vi "SpectrometerSpinCoater_v01.vi"() -> ()   [LabVIEW 2018]
uses:
  <instrlib>/Classes/CCD/Abstract_CCD/Abstract_CCD.lvclass
  TypDef/DeviceQueue_TypeDef.ctl
  TypDef/DeviceQueue_Action.ctl
  TypDef/DataQueue_TypeDef.ctl
  TypDef/DataQueue_Action.ctl
  <vilib>/Utility/error.llb/DialogType.ctl
  <instrlib>/Classes/CCD/Avantes/Avantes.lvclass
  C:/Program Files/National Instruments/LabVIEW 2018/instr.lib/Classes/CCD/Abstract_CCD/Abstract_CCD.lvclass
  <vilib>/Instr/_visa.llb/VISA Configure Serial Port (Instr).vi
panel:
  out "Arduino":bool
  out "NKT":bool
  out "Spectromter":bool
  in  "Abort Button":bool
  in  "Stop Button":bool
  in  "Tab Control":enum32{"Measure", "Settings"}(tab)
  out "Action":string
  in  "Preview":bool
  out "XY Graph":T1(graph)
  in  "Frames for Dark/Ref":dbl=1.0
  in  "StartSpin_Button":bool
  out "Overall Time":dbl
  in  "Seconds after Spin Stop":dbl[unit]=0.5
  in  "Program Spin Coater\nSpeed (rpm)          Time (s)":dbl[][](array[numeric])
  in  "Record RefSpec":bool
  in  "Record_Darkspec":bool
  in  "Comments":string="Just for testing"
  in  "File Name":string="Temp"
  in  "Save Path":path=path "C:/Users/Timo/Desktop/SpinCoater/Measurement"
  in  "Seconds to Spin Start":dbl[unit]=1.0
  in  "Calculate Frames":bool=TRUE
  in  "Frames":i32
  out "Frame Rate":dbl[unit]
  in  "Integration Time":dbl[unit]=3e-05
  in  "StartMeasurement_Button":bool
  in  "Speed":dbl
  in  "Milliseconds":dbl
  in  "Debug":bool
  in  "Port Arduino":refnum<visa-resource-name>="COM3"
  out "Error Arduino":bool caption="Error"
  in  "Init_Arduino":bool=TRUE caption="Init"
  out "Caption_Settings_Arduino":string="Arduino"
  out "Caption_Settings_NKT":string="NKT Laser"
  out "Error_Spectromter":bool caption="Error"
  in  "Init_Spectrometer":bool=TRUE caption="Init"
  out "Caption_Settings_Spectrometer":string="Spectromter"
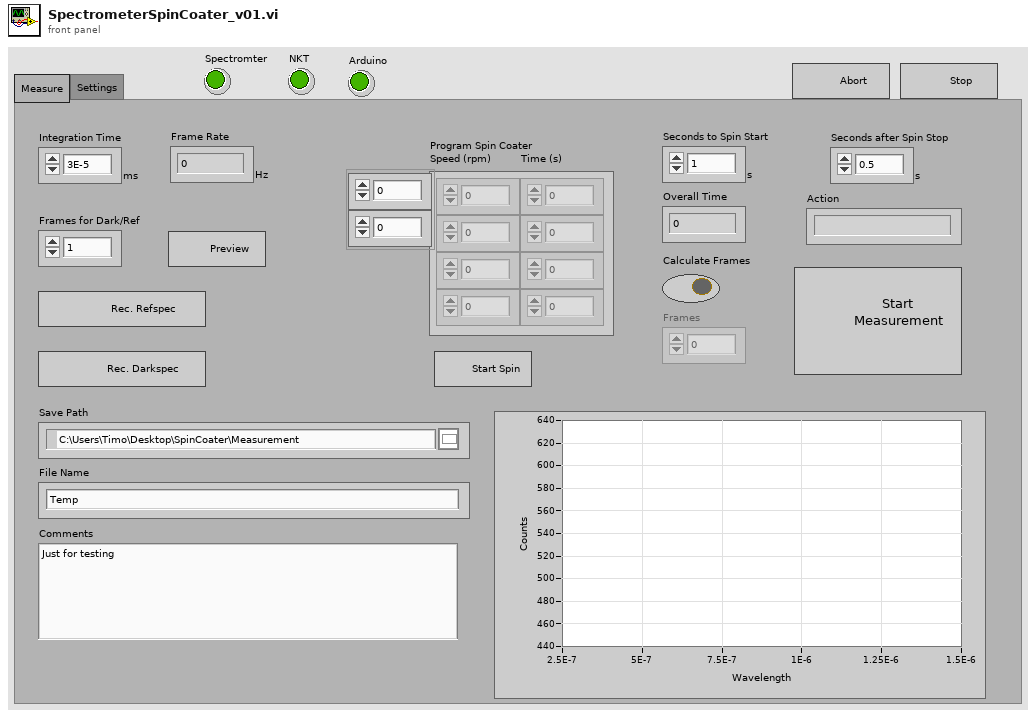
[diagram p1: front panel]
types:
  T1 = cluster{"Wavlength":dbl[unit][], "Image":dbl[]}[]
  T2 = cluster{"Dark":cluster{"Image":dbl[][][], "Frame Size":cluster{"F":i32, "Y":i32, "X":i32}}[], "Ref":cluster{"Image":dbl[][][], "Frame Size":cluster{"F":i32, "Y":i32, "X":i32}}[], "Wavlength":dbl[unit][], "spec":dbl[][]}
  T3 = cluster{"Port Arduino":refnum<visa-resource-name>, "Abstract_CCD.lvclass":refnum<class "Abstract_CCD.lvclass">}
  T4 = typedef "DataQueue_TypeDef.ctl" = cluster{"QueueAction":T5, "Data":cluster{"Image":dbl[][][], "Frame Size":cluster{"F":i32, "Y":i32, "X":i32}}[], "Data_Raw":cluster{"Image":dbl[][][], "Frame Size":cluster{"F":i32, "Y":i32, "X":i32}}[], "Data_Dark":cluster{"Image":dbl[][][], "Frame Size":cluster{"F":i32, "Y":i32, "X":i32}}[], "Data_Ref":cluster{"Image":dbl[][][], "Frame Size":cluster{"F":i32, "Y":i32, "X":i32}}[], "Device Information":string[], "Numeric Control":dbl, "Boolean":bool, "Wavelength":dbl[unit][], "Time":dbl[], "Time Stamp":timestamp}
  T5 = typedef "DataQueue_Action.ctl" = enum16{"TimeOut", "Close_Program", "Measure_InSituSpinCoating", "Save_Data", "Set_Ref", "Set_Dark", "Set_Wavelength", "Spectrometer_Measure"}
  T6 = typedef "DeviceQueue_TypeDef.ctl" = cluster{"QueueAction":T7, "Numeric 1":dbl, "Numeric 2":dbl, "Boolean 1":bool, "Boolean 2":bool, "Spin Program":dbl[][]}
  T7 = typedef "DeviceQueue_Action.ctl" = enum16{"TimeOut", "Close_Program", "Abort", "Spectrometer_Init", "Spectrometer_Close", "Spectrometer_Measure", "Spectrometer_Preview", "Spectrometer_Abort", "Spectrometer_SetIntegrationTime", "Spectrometer_SetFrames", "Spectrometer_SetDarkspec", "Spectrometer_SetReference", "Laser_Init", "Laser_Close", "Arduino_Init", "Arduino_Close", "Arduino_LoadProgram", "Arduino_StartProgram", "Arduino_SetSpeed", "Arduino_SetMillis", "Arduino_StopSpin", "Measure_InSitu"}
  T8 = cluster{"Image":dbl[][][], "Frame Size":cluster{"F":i32, "Y":i32, "X":i32}}[]
  T9 = cluster{"Image":dbl[][][], "Frame Size":cluster{"F":i32, "Y":i32, "X":i32}}
  T10 = cluster{u32, u32, u32, "spec":dbl[][], "Image":dbl[], "Image":dbl[], dbl[], "Time":dbl[], "Numeric Control":dbl}
  T11 = typedef "DialogType.ctl" = u16
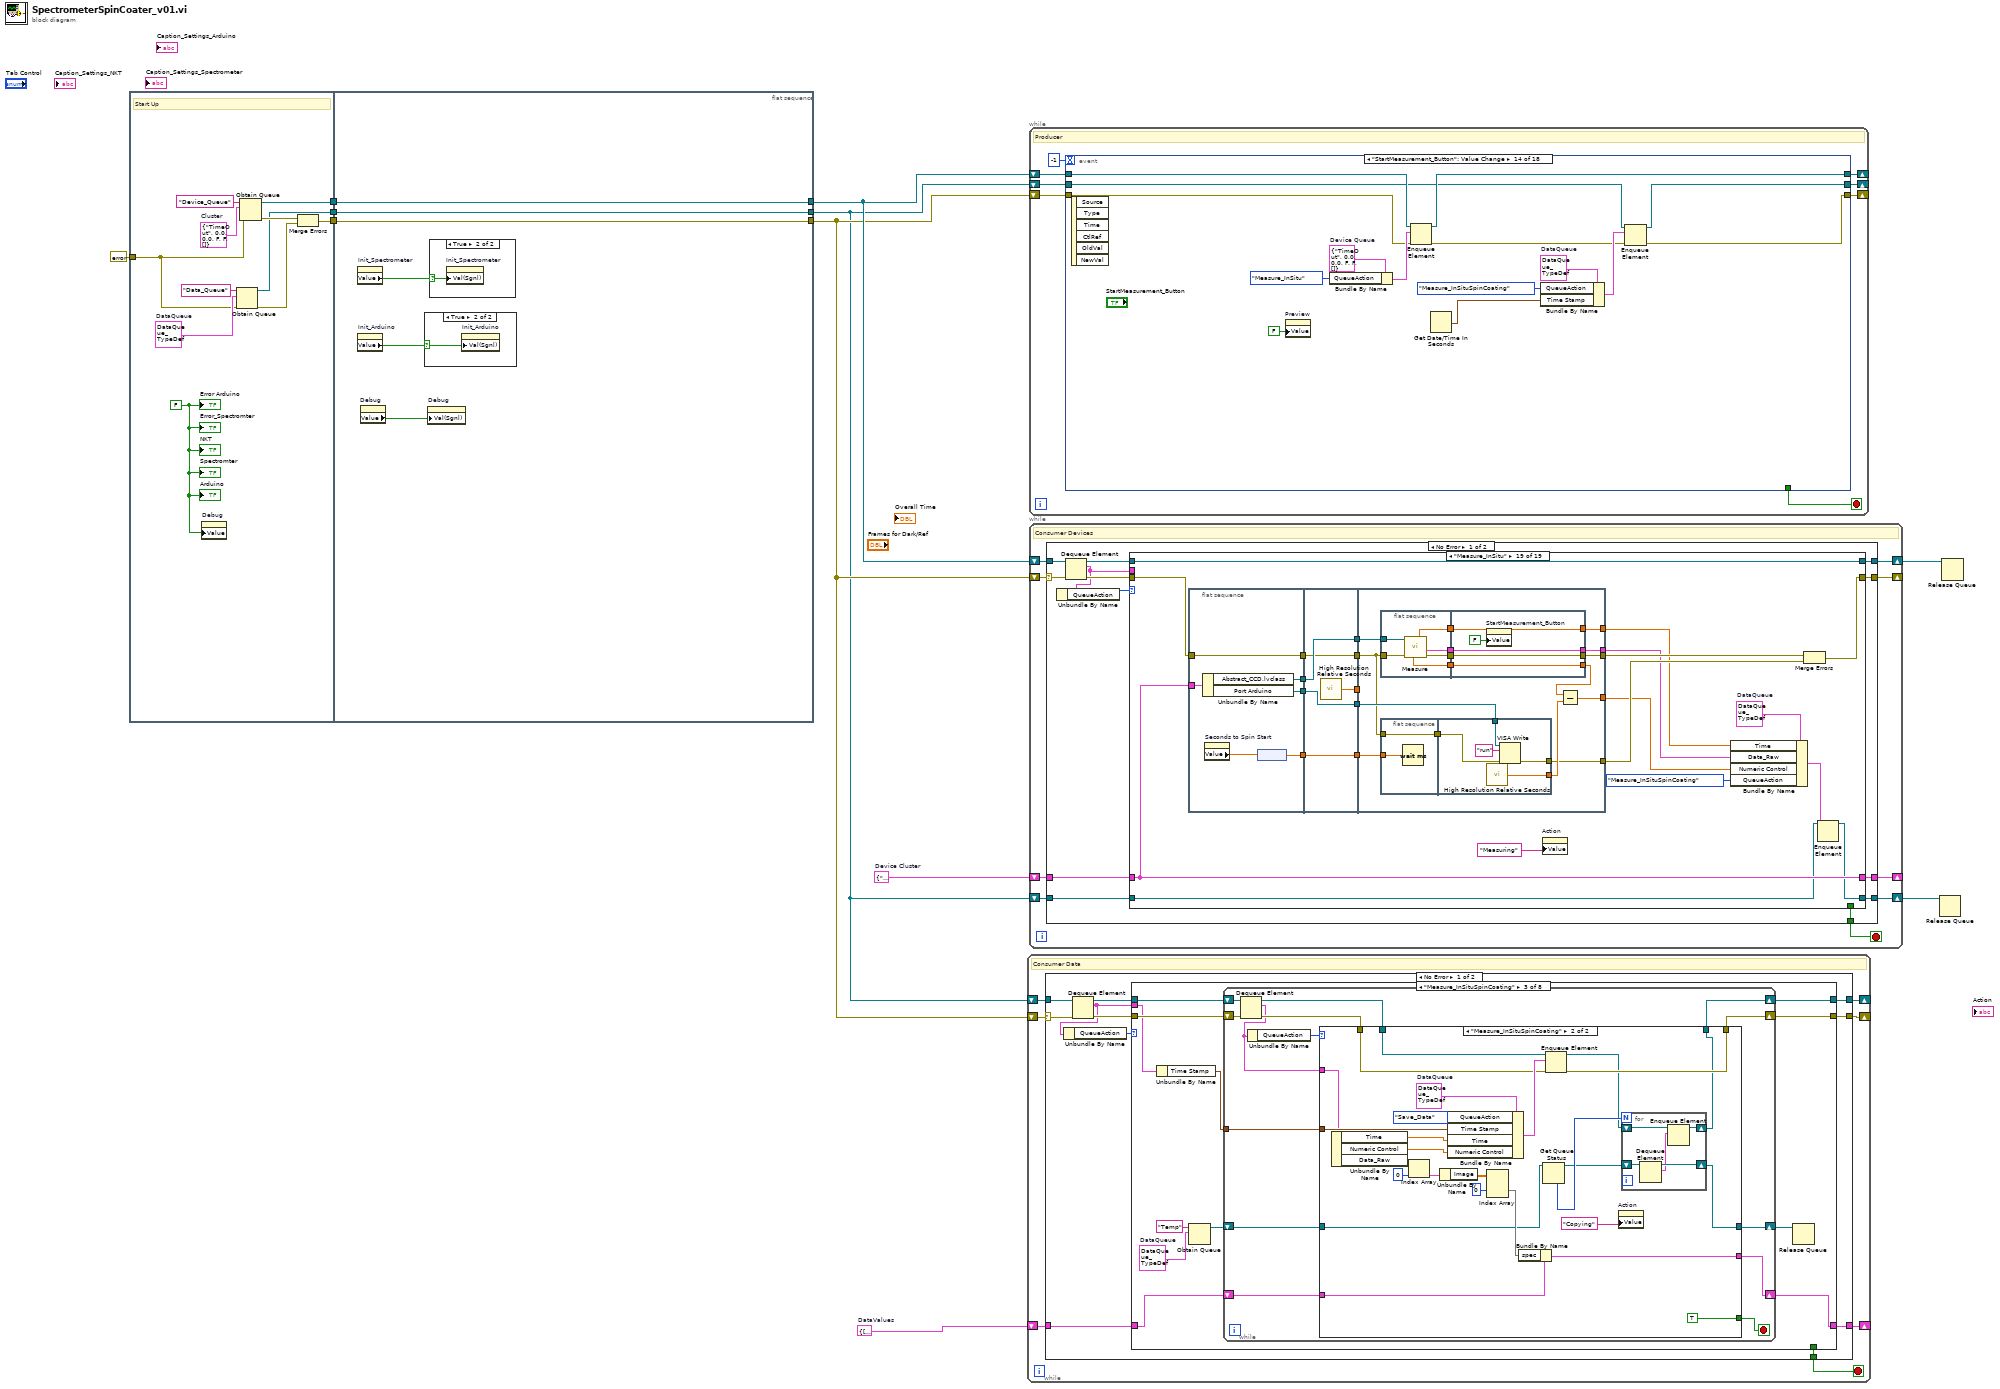
[diagram p0: block diagram]
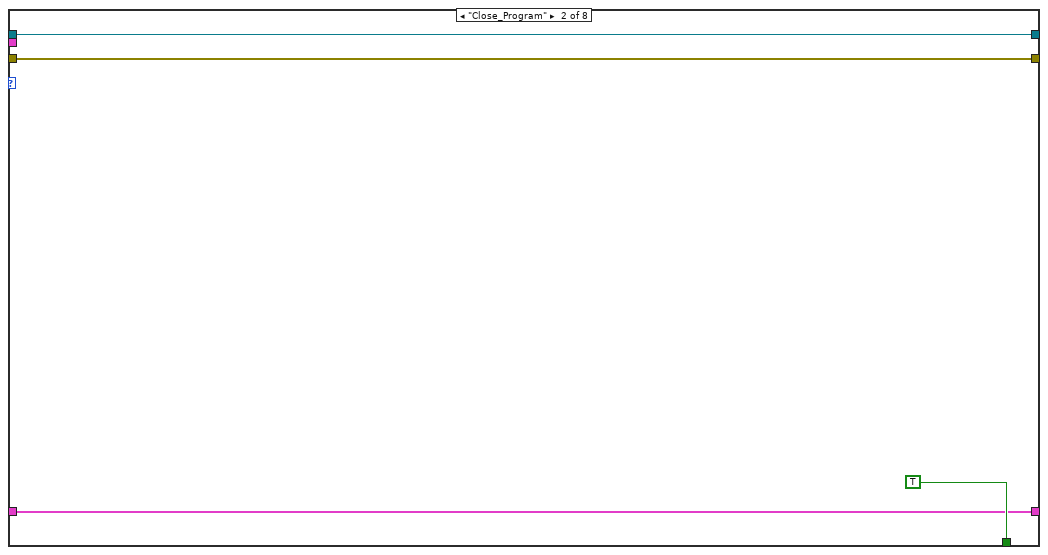
[diagram p5: hidden frame]
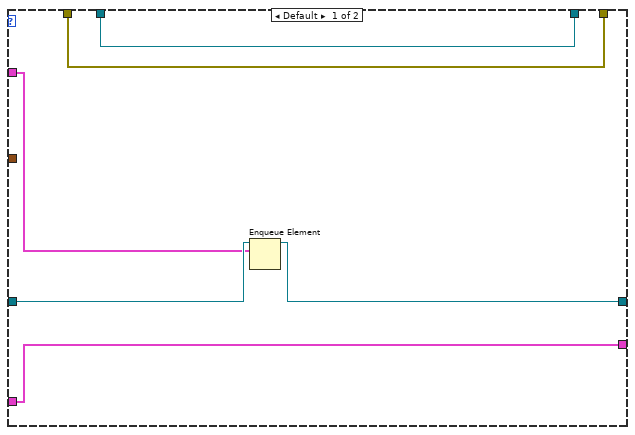
[diagram p6: hidden frame]
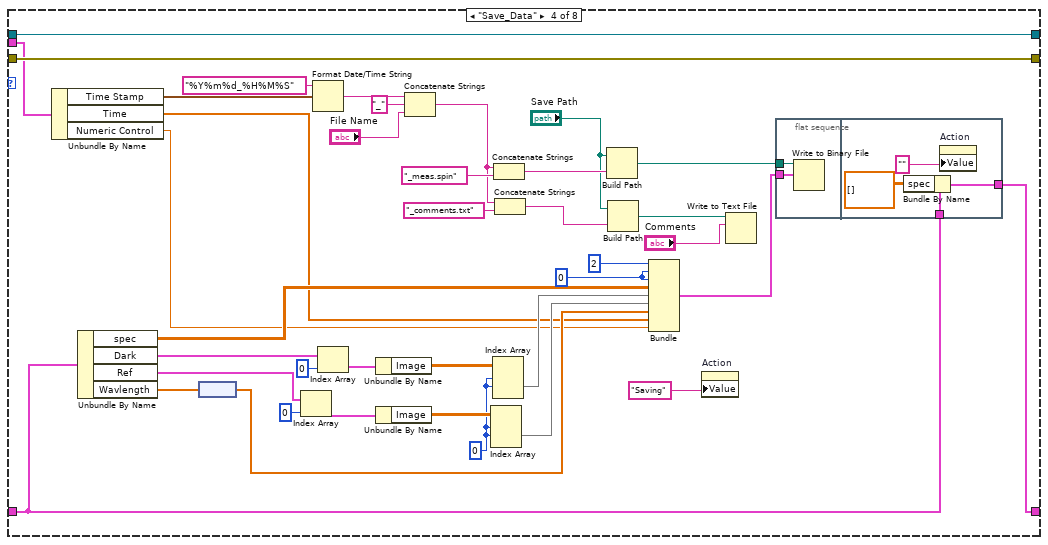
[diagram p7: hidden frame]
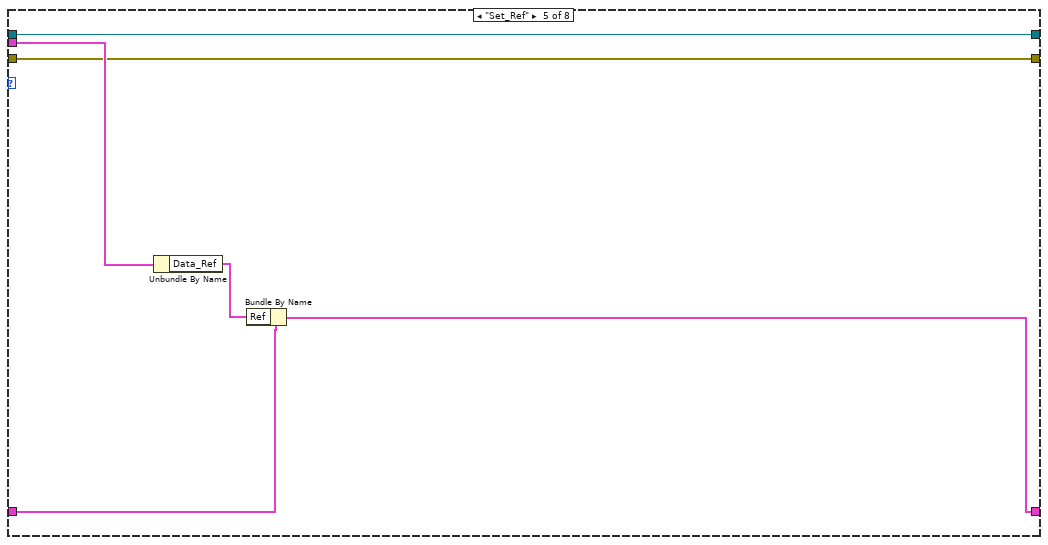
[diagram p8: hidden frame]
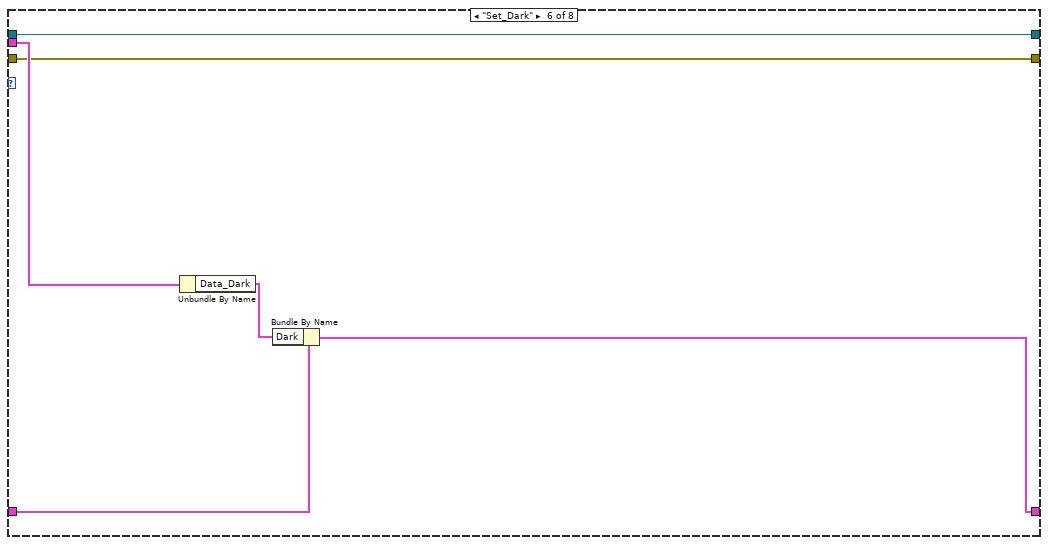
[diagram p9: hidden frame]
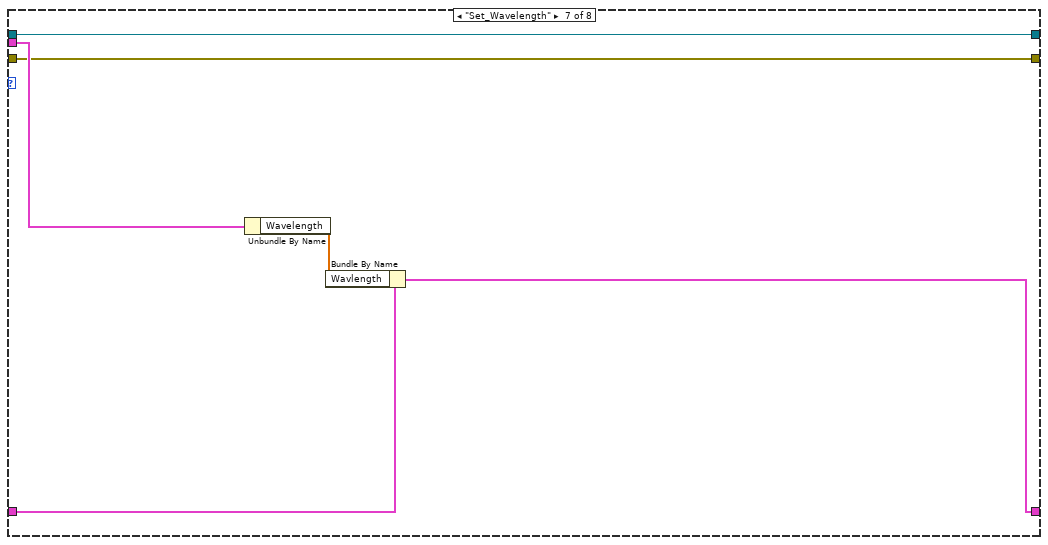
[diagram p10: hidden frame]
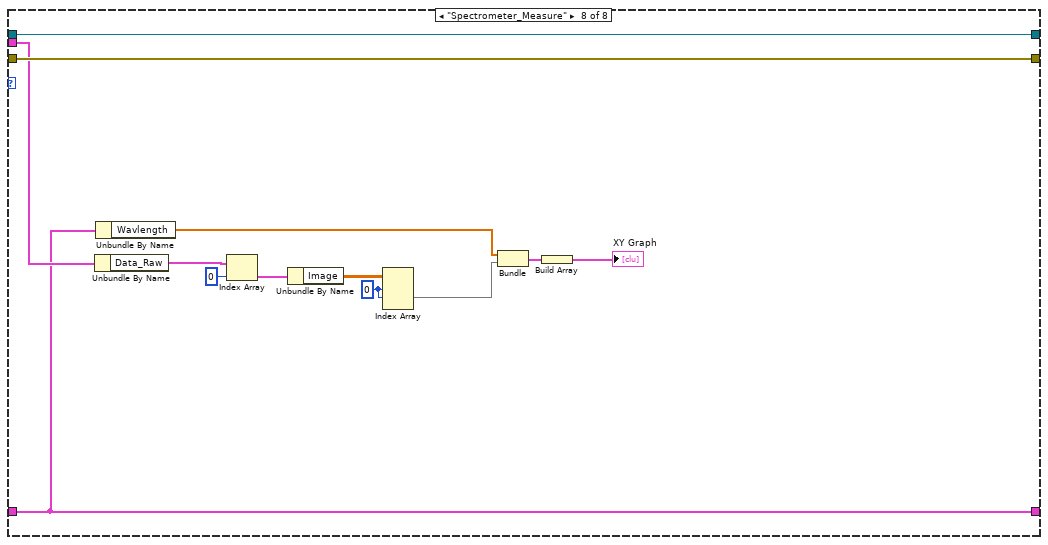
[diagram p11: hidden frame]
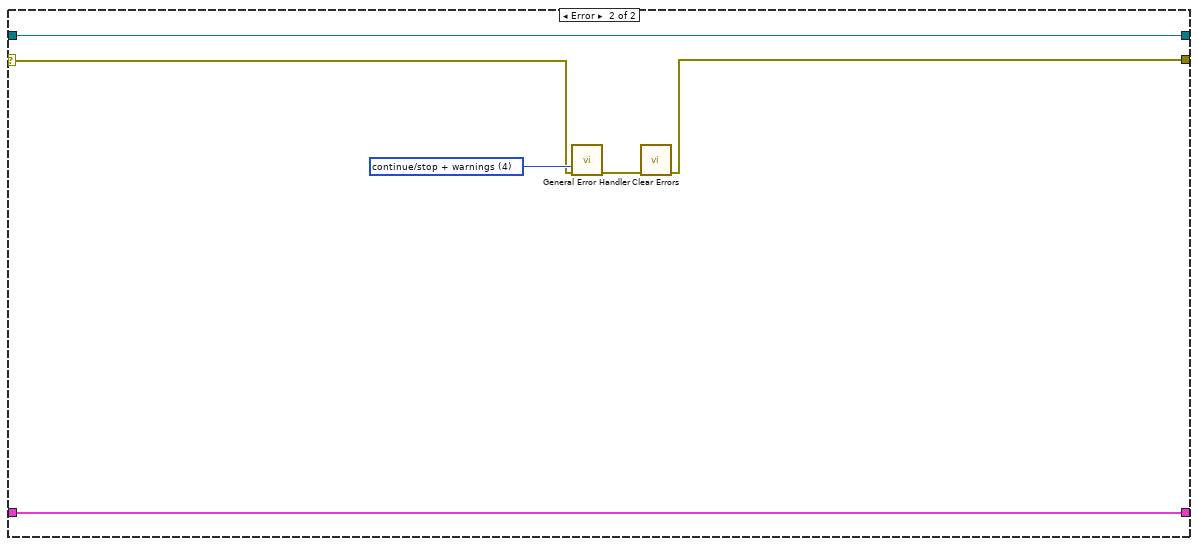
[diagram p12: hidden frame]
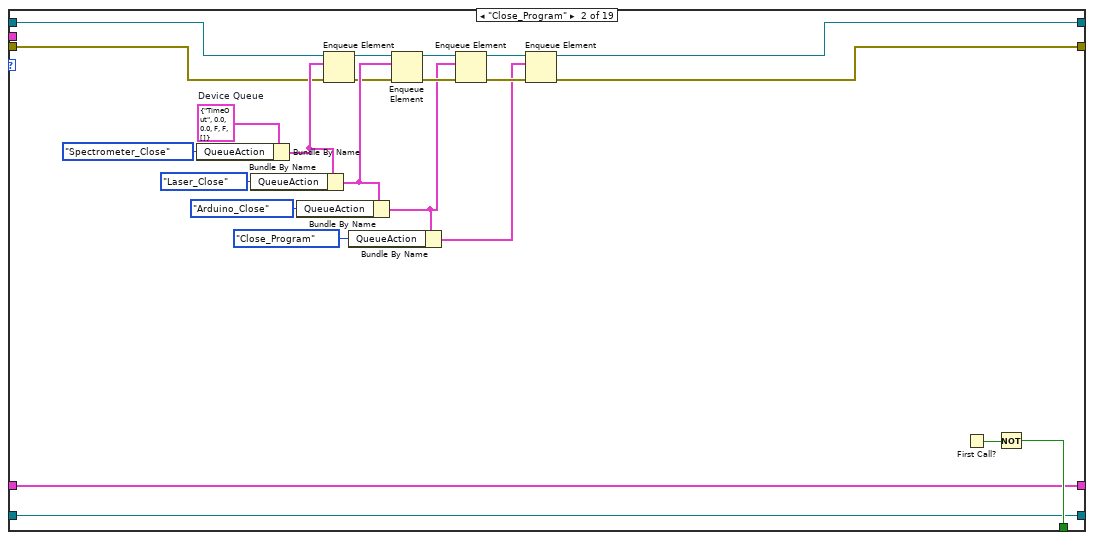
[diagram p14: hidden frame]
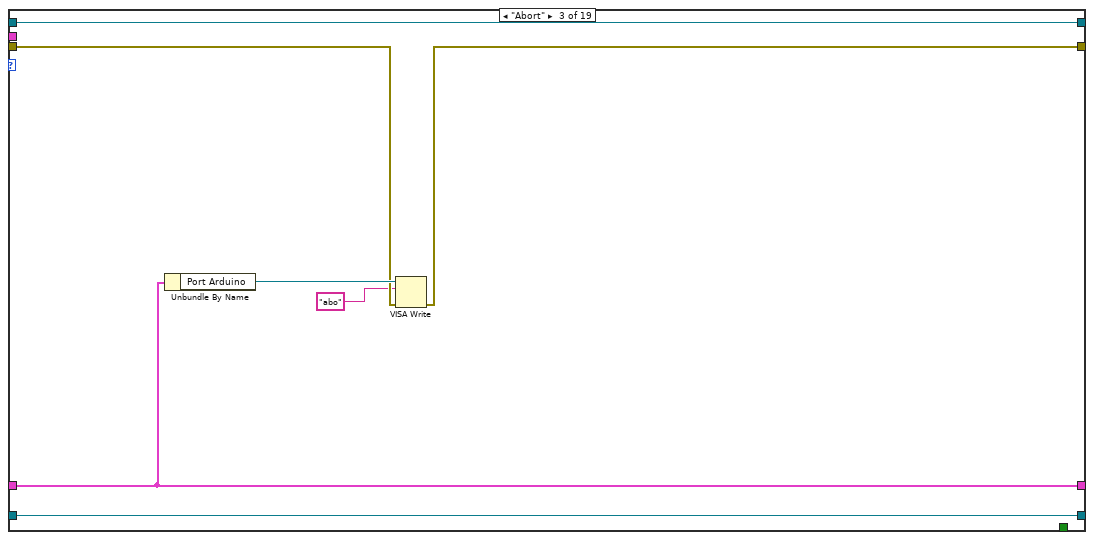
[diagram p15: hidden frame]
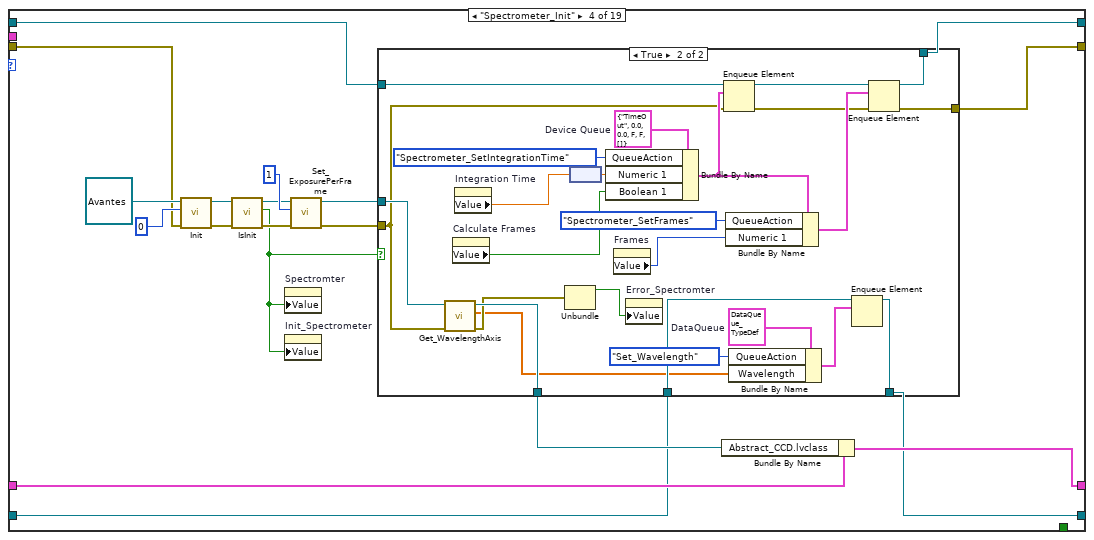
[diagram p16: hidden frame]
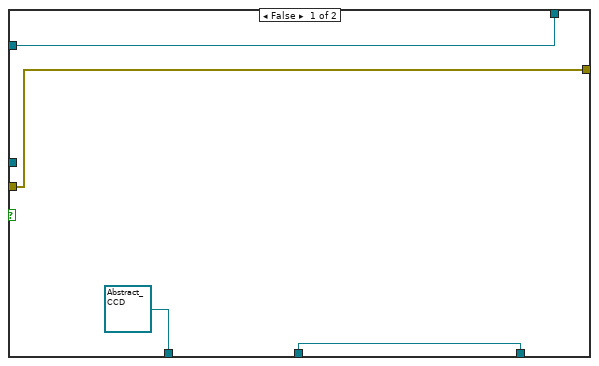
[diagram p17: hidden frame]
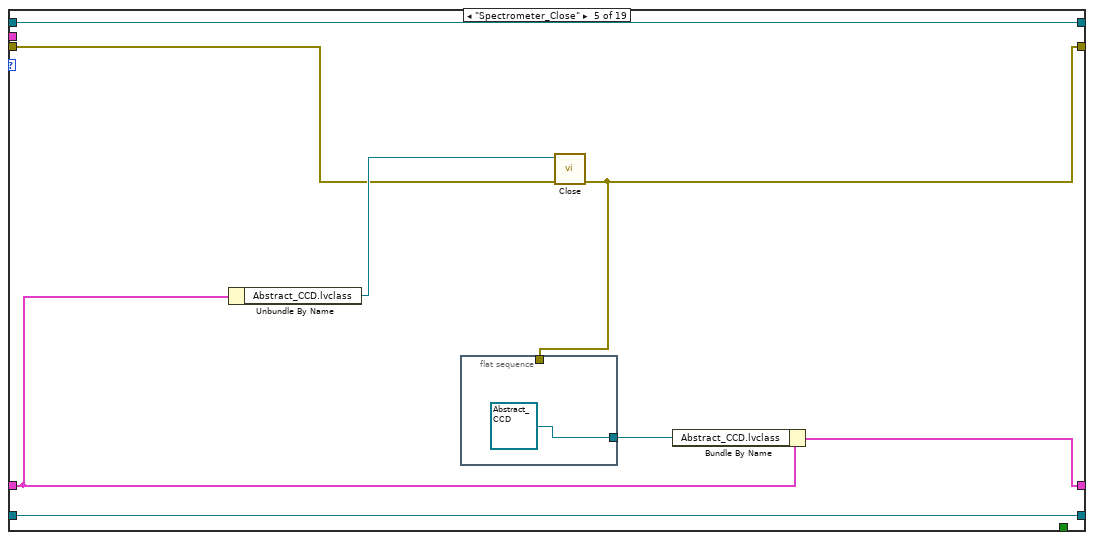
[diagram p18: hidden frame]
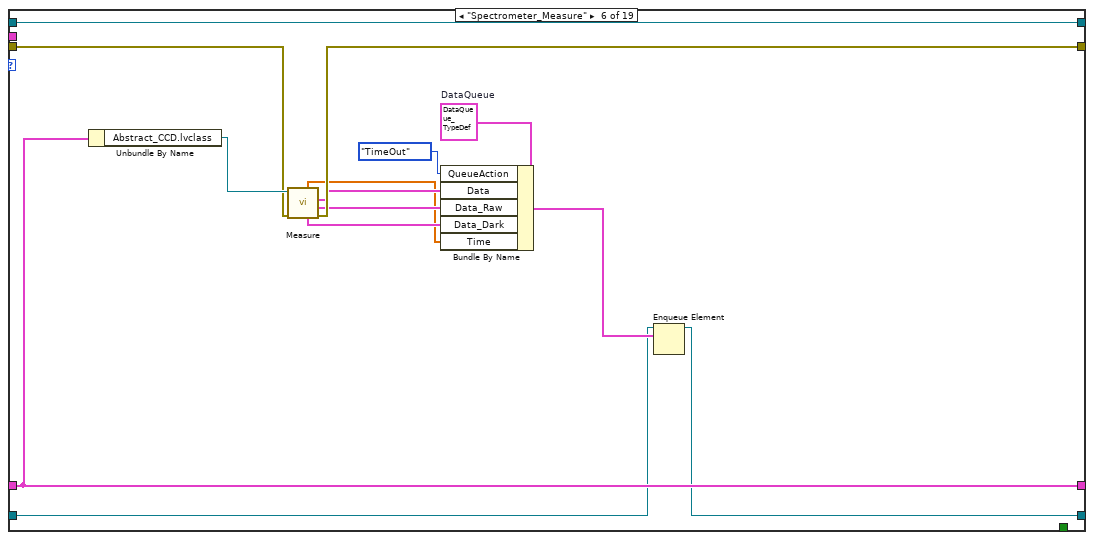
[diagram p19: hidden frame]
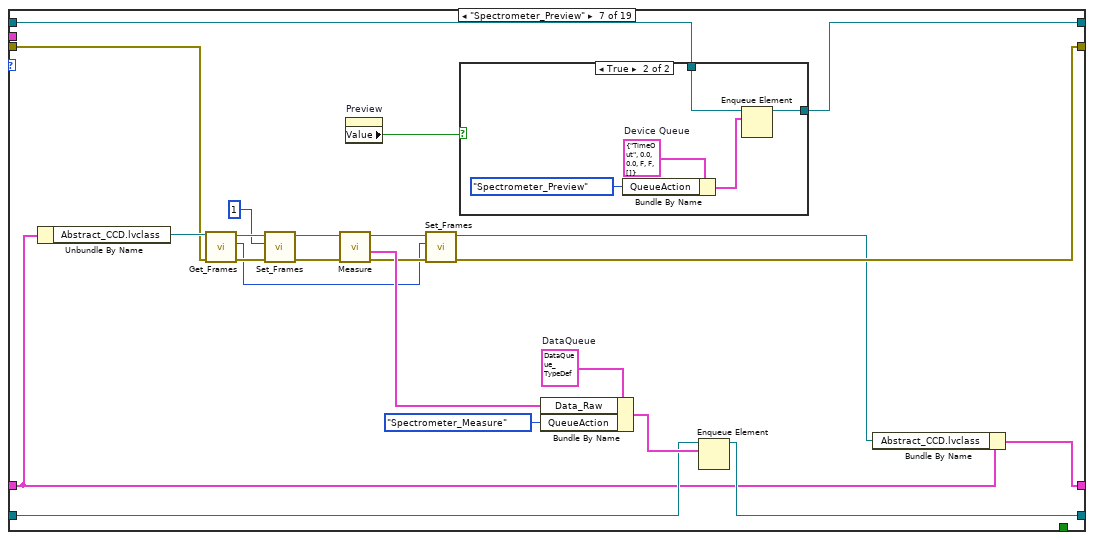
[diagram p20: hidden frame]
diagram:
  w1 = T2 {"Dark"=[], "Ref"=[], "Wavlength"=[], "spec"=[]}  # DataValues
  w6 = T3 {"Port Arduino"="", "Abstract_CCD.lvclass"=refnum}  # Device Cluster
  n1 = flat-sequence {
    tunnel: errorcluster {"status"=FALSE, "code"=0, "source"=""} ("error constant") -> [w17]
    tunnel: [w20] -> w10
    tunnel: [w14] -> w9
    tunnel: [w13] -> w8
    tunnel: w10 -> [w26]
    tunnel: w9 -> [w25]
    tunnel: w8 -> [w24]
    tunnel: [w26] -> w7
    tunnel: [w25] -> w2
    tunnel: [w24] -> w3
    frame #0 {
      w18 = T4 {"QueueAction"=enum."TimeOut", "Data"=[], "Data_Raw"=[], "Data_Dark"=[], "Data_Ref"=[], "Device Information"=[], "Numeric Control"=0.0, "Boolean"=FALSE, "Wavelength"=[], "Time"=[], "Time Stamp"=timestamp(0 s since 1904-01-01)}  # DataQueue
      w21 = T6 {"QueueAction"=enum."TimeOut", "Numeric 1"=0.0, "Numeric 2"=0.0, "Boolean 1"=FALSE, "Boolean 2"=FALSE, "Spin Program"=[]}  # Cluster
      w12 = FALSE ("Error Arduino")
      # "Start Up"
      n2 = property on="Debug" class="Bool (strict)"("Value"=w12) -> ()  [unwired: 2 in, 2 out]
      n3 = Obtain Queue(name (unnamed)="Data_Queue", element data type=w18, error in (no error)=w17) -> (queue out=w14:refnum<queue>, error out=w15:errorcluster)  [unwired: 2 in, 1 out]
      n4 = Obtain Queue(name (unnamed)="Device_Queue", element data type=w21, error in (no error)=w17) -> (queue out=w20:refnum<queue>, error out=w16:errorcluster)  [unwired: 2 in, 1 out]
      n5 = Merge Errors(w16, w15) -> (w13:errorcluster)
      "Error_Spectromter" <- w12
      "Error Arduino" <- w12
      "Spectromter" <- w12
      "NKT" <- w12
      "Arduino" <- w12
    }
    frame #1 {
      n6 = property on="Init_Spectrometer" class="Bool (strict)"() -> ("Value"=w28:bool)  [unwired: 2 in, 2 out]
      n7 = property on="Init_Arduino" class="Bool (strict)"() -> ("Value"=w27:bool)  [unwired: 2 in, 2 out]
      n8 = property on="Debug" class="Bool (strict)"() -> ("Value"=w23:bool)  [unwired: 2 in, 2 out]
      n9 = case shown="True" w27 {
        selector: w27 -> [_ w29]
        frame False {
        }
        frame True {
          n10 = property on="Init_Arduino" class="Bool (strict)"("Val(Sgnl)"=w29) -> ()  [unwired: 2 in, 2 out]
        }
      }
      n11 = property on="Debug" class="Bool (strict)"("Val(Sgnl)"=w23) -> ()  [unwired: 2 in, 2 out]
      n12 = case shown="True" w28 {
        selector: w28 -> [_ w30]
        frame False {
        }
        frame True {
          n13 = property on="Init_Spectrometer" class="Bool (strict)"("Val(Sgnl)"=w30) -> ()  [unwired: 2 in, 2 out]
        }
      }
    }
  }
  n14 = while {
    shift-right: [w31] -> _
    shift-left: w3 -> [w37]
    shift-right: [w32] -> _
    shift-left: w2 -> [w36]
    shift-right: [w33] -> _
    shift-left: w1 -> [w35]
    stop <- w34 stop-if-true
    # "Consumer Data"
    n15 = case shown="No Error" w37 {
      selector: w37 -> [w48 w197]
      tunnel: w36 -> [w47 w198]
      tunnel: w35 -> [w45 w195]
      tunnel: [w44 _] -> w34
      tunnel: [w43 w195] -> w33
      tunnel: [w42 w198] -> w32
      tunnel: [w40 w196] -> w31
      frame No Error {
        n16 = Dequeue Element(queue=w47, error in (no error)=w48) -> (queue out=w41:refnum<queue>, element=w38:T4, error out=w39:errorcluster)  [unwired: 1 in, 1 out]
        n17 = Unbundle By Name(w38) -> ("QueueAction"=w46:T5)
        n18 = case shown="\"Measure_InSituSpinCoating\"" w46 {
          tunnel: w45 -> [w49 w54 w63 w123 w169 w174 w180 w191]
          tunnel: [_ TRUE _ _ _ _ _ _] -> w44
          tunnel: [w49 w54 w59 w122 w168 w170 w179 w191] -> w43
          tunnel: [w51 w53 w67 w157 w167 w171 w176 w194] -> w42
          tunnel: w41 -> [w51 w53 w65 w157 w167 w171 w176 w194]
          tunnel: [w50 w52 w66 w156 w164 w172 w177 w193] -> w40
          tunnel: w39 -> [w50 w52 w64 w156 w164 w172 w177 w193]
          tunnel: w38 -> [_ _ w57 w139 w166 w173 w178 w192]
          frame "TimeOut", Default {
          }
          frame "Close_Program" {
          }
          frame "Measure_InSituSpinCoating" {
            w61 = T4 {"QueueAction"=enum."TimeOut", "Data"=[], "Data_Raw"=[], "Data_Dark"=[], "Data_Ref"=[], "Device Information"=[], "Numeric Control"=0.0, "Boolean"=FALSE, "Wavelength"=[], "Time"=[], "Time Stamp"=timestamp(0 s since 1904-01-01)}  # DataQueue
            n19 = Unbundle By Name(w57) -> ("Time Stamp"=w56:timestamp)
            n20 = Obtain Queue(name (unnamed)="Temp", element data type=w61) -> (queue out=w60:refnum<queue>)  [unwired: 3 in, 2 out]
            n21 = while {
              shift-right: [w81] -> w67
              shift-left: w65 -> [w79]
              shift-right: [w80] -> w66
              shift-left: w64 -> [w78]
              shift-right: [w70] -> w59
              shift-left: w63 -> [w73]
              shift-right: [w71] -> w58
              shift-left: w60 -> [w72]
              tunnel: w56 -> [w69]
              stop <- w68 stop-if-true
              n22 = Dequeue Element(queue=w79, error in (no error)=w78) -> (queue out=w76:refnum<queue>, element=w74:T4, error out=w75:errorcluster)  [unwired: 1 in, 1 out]
              n23 = Unbundle By Name(w74) -> ("QueueAction"=w77:T5)
              n24 = case shown="\"Measure_InSituSpinCoating\"" w77 {
                tunnel: w76 -> [w87 w112]
                tunnel: [w87 w95] -> w81
                tunnel: w75 -> [w86 w111]
                tunnel: [w86 w110] -> w80
                tunnel: [w85 w108] -> w70
                tunnel: w74 -> [w83 w92]
                tunnel: w73 -> [w85 w101]
                tunnel: w72 -> [w84 w100]
                tunnel: [w82 w96] -> w71
                tunnel: w69 -> [_ w94]
                tunnel: [_ TRUE] -> w68
                frame Default {
                  n25 = Enqueue Element(queue=w84, element=w83) -> (queue out=w82:refnum<queue>)  [unwired: 2 in, 2 out]
                }
                frame "Measure_InSituSpinCoating" {
                  w91 = T4 {"QueueAction"=enum."TimeOut", "Data"=[], "Data_Raw"=[], "Data_Dark"=[], "Data_Ref"=[], "Device Information"=[], "Numeric Control"=0.0, "Boolean"=FALSE, "Wavelength"=[], "Time"=[], "Time Stamp"=timestamp(0 s since 1904-01-01)}  # DataQueue
                  n26 = Unbundle By Name(w92) -> ("Time"=w90:dbl[], "Numeric Control"=w89:dbl, "Data_Raw"=w107:T8)
                  n27 = Index Array(array=w107, index=0) -> (element=w105:T9)
                  n28 = Unbundle By Name(w105) -> ("Image"=w104:dbl[][][])
                  n29 = Bundle By Name(cluster=w91, "QueueAction"=DataQueue_Action."Save_Data", "Time Stamp"=w94, "Time"=w90, "Numeric Control"=w89) -> (w113:T4)
                  n30 = Index Array(array=w104, index (dim 1)=0 ("disabled index (row)")) -> (element=w102:dbl[][])  [unwired: 2 in]
                  n31 = Bundle By Name(cluster=w101, "spec"=w102) -> (w108:T2)
                  n32 = Get Queue Status(queue=w100) -> (queue out=w98:refnum<queue>, # elements in queue=w99:i32)  [unwired: 2 in, 6 out]
                  n33 = Enqueue Element(queue=w112, element=w113, error in (no error)=w111) -> (queue out=w97:refnum<queue>, error out=w110:errorcluster)  [unwired: 1 in, 1 out]
                  n34 = property on="Action" class="Str"("Value"="Copying" ("Action")) -> ()  [unwired: 2 in, 2 out]
                  n35 = for {
                    N: w99 -> [_]
                    shift-right: [w117] -> w96
                    shift-left: w98 -> [w118]
                    shift-right: [w114] -> w95
                    shift-left: w97 -> [w115]
                    n36 = Dequeue Element(queue=w118) -> (queue out=w117:refnum<queue>, element=w116:T4)  [unwired: 2 in, 2 out]
                    n37 = Enqueue Element(queue=w115, element=w116) -> (queue out=w114:refnum<queue>)  [unwired: 2 in, 2 out]
                  }
                }
              }
            }
            n38 = Release Queue(queue=w58) -> ()  [unwired: 2 in, 3 out]
          }
          frame "Save_Data" {
            w144 = 0 ("index (page)")
            w155 = u32 0
            n39 = Unbundle By Name(w139) -> ("Time Stamp"=w137:timestamp, "Time"=w121:dbl[], "Numeric Control"=w120:dbl)
            n40 = Unbundle By Name(w123) -> ("spec"=w143:dbl[][], "Dark"=w151:T8, "Ref"=w149:T8, "Wavlength"=w154:dbl[unit][])
            n41 = node(w154) -> (w140:dbl[])
            n42 = Index Array(array=w149, index=0) -> (element=w147:T9)
            n43 = Format Date/Time String(time format string (%c)="%Y%m%d_%H%M%S", seconds (now)=w137) -> (date/time string=w136:string)  [unwired: 1 in]
            n44 = Index Array(array=w151, index=0) -> (element=w148:T9)
            n45 = Unbundle By Name(w148) -> ("Image"=w146:dbl[][][])
            n46 = Unbundle By Name(w147) -> ("Image"=w145:dbl[][][])
            n47 = Concatenate Strings(w136, "_" ("string"), "File Name") -> (w132:string)
            n48 = Index Array(array=w145, index (dim 0)=w144, index (dim 1)=w144) -> (element=w141:dbl[])  [unwired: 1 in]
            n49 = Index Array(array=w146, index (dim 0)=w144, index (dim 1)=w144) -> (element=w142:dbl[])  [unwired: 1 in]
            n50 = Concatenate Strings(w132, "_meas.spin" ("string")) -> (w130:string)
            n51 = Concatenate Strings(w132, "_comments.txt" ("string")) -> (w128:string)
            n52 = Build Path(base path="Save Path", name or relative path=w130) -> (appended path=w124:path)
            n53 = Build Path(base path="Save Path", name or relative path=w128) -> (appended path=w127:path)
            n54 = Bundle(u32 2, w155, w155, "spec"=w143, "Image"=w142, "Image"=w141, w140, "Time"=w121, "Numeric Control"=w120) -> (w125:T10)  [unwired: 1 in]
            n55 = property on="Action" class="Str"("Value"="Saving" ("Action")) -> ()  [unwired: 2 in, 2 out]
            n56 = Write to Text File(file (use dialog)=w127, text="Comments") -> ()  [unwired: 2 in, 3 out]
            n57 = flat-sequence {
              tunnel: w125 -> [w159]
              tunnel: w124 -> [w158]
              tunnel: w123 -> [w163]
              tunnel: [w161] -> w122
              frame #0 {
                n58 = Write to Binary File(file (use dialog)=w158, data=w159) -> ()  [unwired: 4 in, 3 out]
              }
              frame #1 {
                n59 = Bundle By Name(cluster=w163, "spec"=dbl[][] []) -> (w161:T2)
                n60 = property on="Action" class="Str"("Value"="" ("Action")) -> ()  [unwired: 2 in, 2 out]
              }
            }
          }
          frame "Set_Ref" {
            n61 = Unbundle By Name(w166) -> ("Data_Ref"=w165:T8)
            n62 = Bundle By Name(cluster=w169, "Ref"=w165) -> (w168:T2)
          }
          frame "Set_Dark" {
            n63 = Unbundle By Name(w173) -> ("Data_Dark"=w175:T8)
            n64 = Bundle By Name(cluster=w174, "Dark"=w175) -> (w170:T2)
          }
          frame "Set_Wavelength" {
            n65 = Unbundle By Name(w178) -> ("Wavelength"=w181:dbl[unit][])
            n66 = Bundle By Name(cluster=w180, "Wavlength"=w181) -> (w179:T2)
          }
          frame "Spectrometer_Measure" {
            w186 = 0 ("index (page)")
            n67 = Unbundle By Name(w192) -> ("Data_Raw"=w190:T8)
            n68 = Unbundle By Name(w191) -> ("Wavlength"=w185:dbl[unit][])
            n69 = Index Array(array=w190, index=0) -> (element=w188:T9)
            n70 = Unbundle By Name(w188) -> ("Image"=w187:dbl[][][])
            n71 = Index Array(array=w187, index (dim 0)=w186, index (dim 1)=w186) -> (element=w184:dbl[])  [unwired: 1 in]
            n72 = Bundle("Wavlength"=w185, "Image"=w184) -> (w183:cluster{"Wavlength":dbl[unit][], "Image":dbl[]})  [unwired: 1 in]
            n73 = Build Array(w183) -> (→"XY Graph":T1)
          }
        }
      }
      frame Error {
        w200 = T11 4 items=["no dialog", "OK message", "continue or stop message", "OK message + warnings", "continue/stop + warnings"] ("type of dialog (OK msg:1)")
        n74 = call <vilib>:"General Error Handler.vi"("type of dialog (OK msg:1)"=w200, "error in (no error)"=w197) -> ("error out"=w199:errorcluster)  [unwired: 9 in, 4 out]
        n75 = call <vilib>:"Clear Errors.vi"("error in (no error)"=w199) -> ("error out"=w196:errorcluster)  [unwired: 5 in, 1 out]
      }
    }
  }
  n76 = while {
    shift-right: [w203] -> _
    shift-left: w7 -> [w201]
    shift-right: [w206] -> _
    shift-left: w2 -> [w207]
    shift-right: [w204] -> _
    shift-left: w3 -> [w205]
    stop <- w202 stop-if-true
    # "Producer"
    n77 = event shown="[13] \"StartMeasurement_Button\": Value Change" {
      selector: _ -> [_ _ _ _ _ _ _ _ _ _ _ _ _ _ _ _ _ _]
      dyn-events: _ -> [_ _ _ _ _ _ _ _ _ _ _ _ _ _ _ _ _ _]
      timeout: -1 -> [_ _ _ _ _ _ _ _ _ _ _ _ _ _ _ _ _ _]
      tunnel: w207 -> [w210 w225 w229 w241 w254 w267 w279 w290 w292 w300 w319 w326 w335 w343 w358 w368 w377 w385]
      tunnel: [w210 w222 w229 w241 w254 w267 w279 w290 w292 w300 w319 w326 w335 w342 w358 w368 w377 w385] -> w206
      tunnel: w205 -> [w209 w224 w231 w239 w251 w266 w277 w285 w291 w297 w317 w325 w333 w349 w355 w367 w376 w384]
      tunnel: [w209 w218 w228 w235 w250 w264 w275 w284 w291 w295 w316 w323 w332 w341 w356 w364 w373 w384] -> w204
      tunnel: w201 -> [w211 w226 w232 w240 w253 w268 w278 w287 w293 w298 w320 w327 w336 w351 w359 w369 w378 w386]
      tunnel: [w211 w223 w230 w236 w252 w265 w276 w286 w293 w299 w318 w324 w334 w350 w357 w365 w374 w386] -> w203
      tunnel: [_ TRUE _ _ _ _ _ _ _ _ _ _ _ _ _ _ _ _] -> w202
      event Timeout {
        n78 = event-data() -> ()  [unwired: 1 in, 3 out]
      }
      event "Stop Button": Value Change {
        w214 = T4 {"QueueAction"=enum."TimeOut", "Data"=[], "Data_Raw"=[], "Data_Dark"=[], "Data_Ref"=[], "Device Information"=[], "Numeric Control"=0.0, "Boolean"=FALSE, "Wavelength"=[], "Time"=[], "Time Stamp"=timestamp(0 s since 1904-01-01)}  # DataQueue
        w217 = T6 {"QueueAction"=enum."TimeOut", "Numeric 1"=0.0, "Numeric 2"=0.0, "Boolean 1"=FALSE, "Boolean 2"=FALSE, "Spin Program"=[]}  # Device Queue
        n79 = event-data() -> ()  [unwired: 1 in, 6 out]
        n80 = Bundle By Name(cluster=w217, "QueueAction"=DeviceQueue_Action."Close_Program") -> (w215:T6)
        n81 = Enqueue Element(queue=w226, element=w215, error in (no error)=w224) -> (queue out=w223:refnum<queue>, error out=w219:errorcluster)  [unwired: 1 in, 1 out]
        n82 = Bundle By Name(cluster=w214, "QueueAction"=DataQueue_Action."Close_Program") -> (w212:T4)
        n83 = Enqueue Element(queue=w225, element=w212, error in (no error)=w224) -> (queue out=w222:refnum<queue>, error out=w220:errorcluster)  [unwired: 1 in, 1 out]
        n84 = Merge Errors(w220, w219) -> (w218:errorcluster)
      }
      event "Abort Button": Value Change {
        w234 = T6 {"QueueAction"=enum."TimeOut", "Numeric 1"=0.0, "Numeric 2"=0.0, "Boolean 1"=FALSE, "Boolean 2"=FALSE, "Spin Program"=[]}  # Device Queue
        # "At the moment just spin coater in non in-situ measurements can be stopped"
        n85 = event-data() -> ()  [unwired: 1 in, 6 out]
        n86 = Bundle By Name(cluster=w234, "QueueAction"=DeviceQueue_Action."Abort") -> (w233:T6)
        n87 = Enqueue Element(queue=w232, element=w233, error in (no error)=w231) -> (queue out=w230:refnum<queue>, error out=w228:errorcluster)  [unwired: 1 in, 1 out]
      }
      event "Init_Spectrometer": Value Change {
        n88 = event-data() -> ()  [unwired: 1 in, 6 out]
        n89 = case shown="False" "Init_Spectrometer" {
          tunnel: [w242 w245] -> w237
          frame True {
            n90 = Bundle By Name(cluster=T6 {"QueueAction"=enum."TimeOut", "Numeric 1"=0.0, "Numeric 2"=0.0, "Boolean 1"=FALSE, "Boolean 2"=FALSE, "Spin Program"=[]} ("element"), "QueueAction"=DeviceQueue_Action."Spectrometer_Init") -> (w242:T6)
          }
          frame False {
            n91 = Bundle By Name(cluster=T6 {"QueueAction"=enum."TimeOut", "Numeric 1"=0.0, "Numeric 2"=0.0, "Boolean 1"=FALSE, "Boolean 2"=FALSE, "Spin Program"=[]} ("element"), "QueueAction"=DeviceQueue_Action."Spectrometer_Close") -> (w245:T6)
          }
        }
        n92 = Enqueue Element(queue=w240, element=w237, error in (no error)=w239) -> (queue out=w236:refnum<queue>, error out=w235:errorcluster)  [unwired: 1 in, 1 out]
      }
      event "Init_Arduino": Value Change {
        n93 = event-data() -> ("NewVal"=w249:bool)  [unwired: 1 in, 5 out]
        n94 = case shown="True" w249 {
          tunnel: [w255 w258] -> w248
          frame False {
            w257 = T6 {"QueueAction"=enum."TimeOut", "Numeric 1"=0.0, "Numeric 2"=0.0, "Boolean 1"=FALSE, "Boolean 2"=FALSE, "Spin Program"=[]}  # Device Queue
            n95 = Bundle By Name(cluster=w257, "QueueAction"=DeviceQueue_Action."Arduino_Close") -> (w255:T6)
          }
          frame True {
            w260 = T6 {"QueueAction"=enum."TimeOut", "Numeric 1"=0.0, "Numeric 2"=0.0, "Boolean 1"=FALSE, "Boolean 2"=FALSE, "Spin Program"=[]}  # Device Queue
            n96 = Bundle By Name(cluster=w260, "QueueAction"=DeviceQueue_Action."Arduino_Init") -> (w258:T6)
          }
        }
        n97 = Enqueue Element(queue=w253, element=w248, error in (no error)=w251) -> (queue out=w252:refnum<queue>, error out=w250:errorcluster)  [unwired: 1 in, 1 out]
      }
      event "Program Spin Coater\nSpeed (rpm)          Time (s)": Value Change {
        w270 = T6 {"QueueAction"=enum."TimeOut", "Numeric 1"=0.0, "Numeric 2"=0.0, "Boolean 1"=FALSE, "Boolean 2"=FALSE, "Spin Program"=[]}  # Device Queue
        n98 = event-data() -> ("NewVal"=w262:dbl[][])  [unwired: 1 in, 5 out]
        n99 = property on="Integration Time" class="DigNum (strict)"() -> ("Value"=w261:dbl[unit])  [unwired: 2 in, 2 out]
        n100 = property on="Integration Time" class="DigNum (strict)"("Val(Sgnl)"=w261) -> ()  [unwired: 2 in, 2 out]
        n101 = Bundle By Name(cluster=w270, "QueueAction"=DeviceQueue_Action."Arduino_LoadProgram", "Spin Program"=w262) -> (w269:T6)
        n102 = Enqueue Element(queue=w268, element=w269, error in (no error)=w266) -> (queue out=w265:refnum<queue>, error out=w264:errorcluster)  [unwired: 1 in, 1 out]
      }
      event "Integration Time": Value Change {
        w281 = T6 {"QueueAction"=enum."TimeOut", "Numeric 1"=0.0, "Numeric 2"=0.0, "Boolean 1"=FALSE, "Boolean 2"=FALSE, "Spin Program"=[]}  # Device Queue
        n103 = event-data() -> ("NewVal"=w273:dbl[unit])  [unwired: 1 in, 5 out]
        n104 = node(w273) -> (w272:dbl)
        n105 = property on="Calculate Frames" class="Bool (strict)"() -> ("Value"=w271:bool)  [unwired: 2 in, 2 out]
        n106 = Bundle By Name(cluster=w281, "QueueAction"=DeviceQueue_Action."Spectrometer_SetIntegrationTime", "Numeric 1"=w272, "Boolean 1"=w271) -> (w280:T6)
        n107 = Enqueue Element(queue=w278, element=w280, error in (no error)=w277) -> (queue out=w276:refnum<queue>, error out=w275:errorcluster)  [unwired: 1 in, 1 out]
      }
      event "Frames": Value Change {
        w289 = T6 {"QueueAction"=enum."TimeOut", "Numeric 1"=0.0, "Numeric 2"=0.0, "Boolean 1"=FALSE, "Boolean 2"=FALSE, "Spin Program"=[]}  # Device Queue
        n108 = event-data() -> ()  [unwired: 1 in, 6 out]
        n109 = Bundle By Name(cluster=w289, "QueueAction"=DeviceQueue_Action."Spectrometer_SetFrames", "Numeric 1"="Frames") -> (w288:T6)
        n110 = Enqueue Element(queue=w287, element=w288, error in (no error)=w285) -> (queue out=w286:refnum<queue>, error out=w284:errorcluster)  [unwired: 1 in, 1 out]
      }
      event "Seconds to Spin Start", "Seconds after Spin Stop": Value Change {
        n111 = event-data() -> ()  [unwired: 1 in, 6 out]
        n112 = property on="Integration Time" class="DigNum (strict)"() -> ("Value"=w294:dbl[unit])  [unwired: 2 in, 2 out]
        n113 = property on="Integration Time" class="DigNum (strict)"("Val(Sgnl)"=w294) -> ()  [unwired: 2 in, 2 out]
      }
      event "Calculate Frames": Value Change {
        n114 = event-data() -> ("NewVal"=w301:bool)  [unwired: 1 in, 5 out]
        n115 = case shown="False" w301 {
          tunnel: [0 2] -> w296
          tunnel: w298 -> [w303 w312]
          tunnel: [w303 w310] -> w299
          tunnel: w297 -> [w302 w309]
          tunnel: [w302 w305] -> w295
          frame False {
          }
          frame True {
            w311 = T6 {"QueueAction"=enum."TimeOut", "Numeric 1"=0.0, "Numeric 2"=0.0, "Boolean 1"=FALSE, "Boolean 2"=FALSE, "Spin Program"=[]}  # Device Queue
            n116 = property on="Integration Time" class="DigNum (strict)"() -> ("Value"=w307:dbl[unit])  [unwired: 2 in, 2 out]
            n117 = node(w307) -> (w306:dbl)
            n118 = Bundle By Name(cluster=w311, "QueueAction"=DeviceQueue_Action."Spectrometer_SetIntegrationTime", "Numeric 1"=w306) -> (w313:T6)
            n119 = Enqueue Element(queue=w312, element=w313, error in (no error)=w309) -> (queue out=w310:refnum<queue>, error out=w305:errorcluster)  [unwired: 1 in, 1 out]
          }
        }
        n120 = property on="Frames" class="DigNum (strict)"("DisabledEnum"=w296) -> ()  [unwired: 2 in, 2 out]
      }
      event "Record RefSpec": Value Change {
        w322 = T6 {"QueueAction"=enum."TimeOut", "Numeric 1"=0.0, "Numeric 2"=0.0, "Boolean 1"=FALSE, "Boolean 2"=FALSE, "Spin Program"=[]}  # Device Queue
        n121 = event-data() -> ()  [unwired: 1 in, 6 out]
        n122 = Bundle By Name(cluster=w322, "QueueAction"=DeviceQueue_Action."Spectrometer_SetReference") -> (w321:T6)
        n123 = Enqueue Element(queue=w320, element=w321, error in (no error)=w317) -> (queue out=w318:refnum<queue>, error out=w316:errorcluster)  [unwired: 1 in, 1 out]
      }
      event "Preview": Value Change {
        w330 = T6 {"QueueAction"=enum."TimeOut", "Numeric 1"=0.0, "Numeric 2"=0.0, "Boolean 1"=FALSE, "Boolean 2"=FALSE, "Spin Program"=[]}  # Device Queue
        n124 = event-data() -> ()  [unwired: 1 in, 6 out]
        n125 = Bundle By Name(cluster=w330, "QueueAction"=DeviceQueue_Action."Spectrometer_Preview") -> (w329:T6)
        n126 = Enqueue Element(queue=w327, element=w329, error in (no error)=w325) -> (queue out=w324:refnum<queue>, error out=w323:errorcluster)  [unwired: 1 in, 1 out]
      }
      event "Record_Darkspec": Value Change {
        w338 = T6 {"QueueAction"=enum."TimeOut", "Numeric 1"=0.0, "Numeric 2"=0.0, "Boolean 1"=FALSE, "Boolean 2"=FALSE, "Spin Program"=[]}  # Device Queue
        n127 = event-data() -> ()  [unwired: 1 in, 6 out]
        n128 = Bundle By Name(cluster=w338, "QueueAction"=DeviceQueue_Action."Spectrometer_SetDarkspec") -> (w337:T6)
        n129 = Enqueue Element(queue=w336, element=w337, error in (no error)=w333) -> (queue out=w334:refnum<queue>, error out=w332:errorcluster)  [unwired: 1 in, 1 out]
      }
      event "StartMeasurement_Button": Value Change {
        w345 = T4 {"QueueAction"=enum."TimeOut", "Data"=[], "Data_Raw"=[], "Data_Dark"=[], "Data_Ref"=[], "Device Information"=[], "Numeric Control"=0.0, "Boolean"=FALSE, "Wavelength"=[], "Time"=[], "Time Stamp"=timestamp(0 s since 1904-01-01)}  # DataQueue
        w353 = T6 {"QueueAction"=enum."TimeOut", "Numeric 1"=0.0, "Numeric 2"=0.0, "Boolean 1"=FALSE, "Boolean 2"=FALSE, "Spin Program"=[]}  # Device Queue
        n130 = event-data() -> ()  [unwired: 1 in, 6 out]
        n131 = property on="Preview" class="Bool (strict)"("Value"=FALSE ("Preview")) -> ()  [unwired: 2 in, 2 out]
        n132 = Bundle By Name(cluster=w353, "QueueAction"=DeviceQueue_Action."Measure_InSitu") -> (w352:T6)
        n133 = Enqueue Element(queue=w351, element=w352, error in (no error)=w349) -> (queue out=w350:refnum<queue>, error out=w340:errorcluster)  [unwired: 1 in, 1 out]
        n134 = Get Date/Time In Seconds() -> (seconds since 1Jan1904=w339:timestamp)
        n135 = Bundle By Name(cluster=w345, "QueueAction"=DataQueue_Action."Measure_InSituSpinCoating", "Time Stamp"=w339) -> (w346:T4)
        n136 = Enqueue Element(queue=w343, element=w346, error in (no error)=w340) -> (queue out=w342:refnum<queue>, error out=w341:errorcluster)  [unwired: 1 in, 1 out]
      }
      event "StartSpin_Button": Value Change {
        w361 = T6 {"QueueAction"=enum."TimeOut", "Numeric 1"=0.0, "Numeric 2"=0.0, "Boolean 1"=FALSE, "Boolean 2"=FALSE, "Spin Program"=[]}  # Device Queue
        n137 = event-data() -> ()  [unwired: 1 in, 6 out]
        n138 = Bundle By Name(cluster=w361, "QueueAction"=DeviceQueue_Action."Arduino_StartProgram") -> (w360:T6)
        n139 = Enqueue Element(queue=w359, element=w360, error in (no error)=w355) -> (queue out=w357:refnum<queue>, error out=w356:errorcluster)  [unwired: 1 in, 1 out]
      }
      event "Milliseconds": Value Change {
        w370 = T6 {"QueueAction"=enum."TimeOut", "Numeric 1"=0.0, "Numeric 2"=0.0, "Boolean 1"=FALSE, "Boolean 2"=FALSE, "Spin Program"=[]}  # Device Queue
        n140 = event-data() -> ()  [unwired: 1 in, 6 out]
        n141 = Bundle By Name(cluster=w370, "QueueAction"=DeviceQueue_Action."Arduino_SetMillis", "Numeric 1"="Milliseconds") -> (w366:T6)
        n142 = Enqueue Element(queue=w369, element=w366, error in (no error)=w367) -> (queue out=w365:refnum<queue>, error out=w364:errorcluster)  [unwired: 1 in, 1 out]
      }
      event "Speed": Value Change {
        w379 = T6 {"QueueAction"=enum."TimeOut", "Numeric 1"=0.0, "Numeric 2"=0.0, "Boolean 1"=FALSE, "Boolean 2"=FALSE, "Spin Program"=[]}  # Device Queue
        n143 = event-data() -> ()  [unwired: 1 in, 6 out]
        n144 = Bundle By Name(cluster=w379, "QueueAction"=DeviceQueue_Action."Arduino_SetSpeed", "Numeric 1"="Speed") -> (w375:T6)
        n145 = Enqueue Element(queue=w378, element=w375, error in (no error)=w376) -> (queue out=w374:refnum<queue>, error out=w373:errorcluster)  [unwired: 1 in, 1 out]
      }
      event "Debug": Value Change {
        n146 = event-data() -> ()  [unwired: 1 in, 6 out]
        n147 = Select(t=u8 0, s="Debug", f=u8 2) -> (s? t:f=w380:u8)
        n148 = property on="Milliseconds" class="DigNum (strict)"("DisabledEnum"=w380) -> ()  [unwired: 2 in, 2 out]
        n149 = property on="Speed" class="DigNum (strict)"("DisabledEnum"=w380) -> ()  [unwired: 2 in, 2 out]
      }
    }
  }
  n150 = while {
    shift-right: [w391] -> _
    shift-left: w3 -> [w395]
    shift-right: [w392] -> w5
    shift-left: w7 -> [w394]
    shift-right: [w389] -> w4
    shift-left: w2 -> [w390]
    shift-right: [w387] -> _
    shift-left: w6 -> [w388]
    stop <- w393 stop-if-true
    # "Consumer Devices"
    n151 = case shown="No Error" w395 {
      selector: w395 -> [w407 w769]
      tunnel: w394 -> [w408 w770]
      tunnel: [w404 _] -> w393
      tunnel: [w403 w770] -> w392
      tunnel: [w401 w766] -> w391
      tunnel: w390 -> [w399 w764]
      tunnel: [w400 w764] -> w389
      tunnel: w388 -> [w398 w765]
      tunnel: [w397 w765] -> w387
      frame No Error {
        n152 = Dequeue Element(queue=w408, error in (no error)=w407) -> (queue out=w406:refnum<queue>, element=w396:T6, error out=w402:errorcluster)  [unwired: 1 in, 1 out]
        n153 = Unbundle By Name(w396) -> ("QueueAction"=w405:T7)
        n154 = case shown="\"Measure_InSitu\"" w405 {
          tunnel: w406 -> [w412 w432 w438 w447 w496 w510 w517 w548 w578 w601 w622 w631 w642 w656 w657 w664 w680 w693 w718]
          tunnel: [_ w434 _ _ _ _ _ _ _ _ _ _ _ _ _ _ _ _ _] -> w404
          tunnel: [w412 w417 w438 w446 w496 w510 w518 w547 w578 w601 w622 w624 w642 w656 w657 w664 w680 w693 w718] -> w403
          tunnel: w402 -> [w411 w416 w439 w458 w497 w509 w532 w554 w576 w592 w613 w640 w646 w655 w659 w671 w681 w692 w709]
          tunnel: [w411 w415 w437 w445 w491 w508 w519 w546 w575 w591 w612 w623 w645 w651 w658 w665 w679 w688 w706] -> w401
          tunnel: [w409 w414 w442 w443 w493 w505 w526 w556 w579 w584 w605 w638 w644 w653 w663 w675 w677 w694 w696] -> w400
          tunnel: w399 -> [w409 w414 w442 w444 w493 w506 w527 w556 w579 w587 w608 w638 w644 w653 w663 w675 w677 w694 w697]
          tunnel: w398 -> [w410 w413 w441 w455 w495 w507 w516 w545 w572 w583 w604 w637 w643 w652 w662 w674 w676 w691 w704]
          tunnel: [w410 w413 w441 w449 w494 w507 w515 w543 w573 w582 w603 w635 w643 w652 w662 w674 w676 w691 w704] -> w397
          tunnel: w396 -> [_ _ _ _ _ _ _ w551 w580 _ _ _ _ w650 _ w672 w678 _ _]
          frame "TimeOut", Default {
          }
          frame "Close_Program" {
            w433 = T6 {"QueueAction"=enum."TimeOut", "Numeric 1"=0.0, "Numeric 2"=0.0, "Boolean 1"=FALSE, "Boolean 2"=FALSE, "Spin Program"=[]}  # Device Queue
            n155 = Bundle By Name(cluster=w433, "QueueAction"=DeviceQueue_Action."Spectrometer_Close") -> (w428:T6)
            n156 = Bundle By Name(cluster=w428, "QueueAction"=DeviceQueue_Action."Laser_Close") -> (w426:T6)
            n157 = Bundle By Name(cluster=w426, "QueueAction"=DeviceQueue_Action."Arduino_Close") -> (w420:T6)
            n158 = Enqueue Element(queue=w432, element=w428, error in (no error)=w416) -> (queue out=w430:refnum<queue>, error out=w425:errorcluster)  [unwired: 1 in, 1 out]
            n159 = Bundle By Name(cluster=w420, "QueueAction"=DeviceQueue_Action."Close_Program") -> (w418:T6)
            n160 = Enqueue Element(queue=w430, element=w426, error in (no error)=w425) -> (queue out=w424:refnum<queue>, error out=w423:errorcluster)  [unwired: 1 in, 1 out]
            n161 = Enqueue Element(queue=w424, element=w420, error in (no error)=w423) -> (queue out=w422:refnum<queue>, error out=w421:errorcluster)  [unwired: 1 in, 1 out]
            n162 = Enqueue Element(queue=w422, element=w418, error in (no error)=w421) -> (queue out=w417:refnum<queue>, error out=w415:errorcluster)  [unwired: 1 in, 1 out]
            n163 = First Call?() -> (First Call?: T/F=w435:bool)
            n164 = Not(x=w435) -> (.not. x?=w434:bool)
          }
          frame "Abort" {
            n165 = Unbundle By Name(w441) -> ("Port Arduino"=w440:refnum<visa-resource-name>)
            n166 = VISA Write(VISA resource name=w440, write buffer="abo", error in (no error)=w439) -> (error out=w437:errorcluster)  [unwired: 2 out]
          }
          frame "Spectrometer_Init" {
            n167 = call-dynamic "Init.vi"("error in (no error)"=w458, "Variant"=0, "Avantes in"=refnum<class "Avantes.lvclass"> refnum ("Avantes.lvclass")) -> ("error out"=w457:errorcluster, "Avantes out"=w456:refnum<class "Avantes.lvclass">)  [unwired: 7 in]
            n168 = call-dynamic "IsInit.vi"("error in (no error)"=w457, "Avantes in"=w456) -> ("error out"=w453:errorcluster, "Is Init?"=w452:bool, "Avantes out"=w454:refnum<class "Avantes.lvclass">)  [unwired: 7 in]
            n169 = property on="Spectromter" class="Bool (strict)"("Value"=w452) -> ()  [unwired: 2 in, 2 out]
            n170 = property on="Init_Spectrometer" class="Bool (strict)"("Value"=w452) -> ()  [unwired: 2 in, 2 out]
            n171 = call-dynamic "Set_ExposurePerFrame.vi"("error in (no error)"=w453, "Exposure per Frame"=1, "Avantes in"=w454) -> ("error out"=w448:errorcluster, "Avantes out"=w451:refnum<class "Avantes.lvclass">)  [unwired: 7 in]
            n172 = case shown="True" w452 {
              tunnel: w451 -> [_ w474]
              tunnel: w448 -> [w463 w472]
              tunnel: [refnum<class "Abstract_CCD.lvclass"> refnum ("Abstract_CCD.lvclass") w473] -> w450
              tunnel: w447 -> [w464 w489]
              tunnel: [w464 w478] -> w446
              tunnel: [w463 w477] -> w445
              tunnel: w444 -> [w462 w469]
              tunnel: [w462 w467] -> w443
              frame False {
              }
              frame True {
                w475 = T4 {"QueueAction"=enum."TimeOut", "Data"=[], "Data_Raw"=[], "Data_Dark"=[], "Data_Ref"=[], "Device Information"=[], "Numeric Control"=0.0, "Boolean"=FALSE, "Wavelength"=[], "Time"=[], "Time Stamp"=timestamp(0 s since 1904-01-01)}  # DataQueue
                w490 = T6 {"QueueAction"=enum."TimeOut", "Numeric 1"=0.0, "Numeric 2"=0.0, "Boolean 1"=FALSE, "Boolean 2"=FALSE, "Spin Program"=[]}  # Device Queue
                n173 = call-dynamic "Get_WavelengthAxis.vi"("error in (no error)"=w472, "Avantes in"=w474) -> ("error out"=w471:errorcluster, "lambda"=w466:dbl[unit][], "Avantes out"=w473:refnum<class "Avantes.lvclass">)  [unwired: 7 in]
                n174 = property on="Calculate Frames" class="Bool (strict)"() -> ("Value"=w482:bool)  [unwired: 2 in, 2 out]
                n175 = property on="Integration Time" class="DigNum (strict)"() -> ("Value"=w487:dbl[unit])  [unwired: 2 in, 2 out]
                n176 = Unbundle(w471) -> ("status"=w470:bool)  [unwired: 2 out]
                n177 = node(w487) -> (w486:dbl)
                n178 = Bundle By Name(cluster=w490, "QueueAction"=DeviceQueue_Action."Spectrometer_SetIntegrationTime", "Numeric 1"=w486, "Boolean 1"=w482) -> (w484:T6)
                n179 = property on="Frames" class="DigNum (strict)"() -> ("Value"=w481:i32)  [unwired: 2 in, 2 out]
                n180 = property on="Error_Spectromter" class="Bool (strict)"("Value"=w470) -> ()  [unwired: 2 in, 2 out]
                n181 = Enqueue Element(queue=w489, element=w484, error in (no error)=w472) -> (queue out=w485:refnum<queue>, error out=w479:errorcluster)  [unwired: 1 in, 1 out]
                n182 = Bundle By Name(cluster=w484, "QueueAction"=DeviceQueue_Action."Spectrometer_SetFrames", "Numeric 1"=w481) -> (w480:T6)
                n183 = Bundle By Name(cluster=w475, "QueueAction"=DataQueue_Action."Set_Wavelength", "Wavelength"=w466) -> (w476:T4)
                n184 = Enqueue Element(queue=w469, element=w476) -> (queue out=w467:refnum<queue>)  [unwired: 2 in, 2 out]
                n185 = Enqueue Element(queue=w485, element=w480, error in (no error)=w479) -> (queue out=w478:refnum<queue>, error out=w477:errorcluster)  [unwired: 1 in, 1 out]
              }
            }
            n186 = Bundle By Name(cluster=w455, "Abstract_CCD.lvclass"=w450) -> (w449:T3)
          }
          frame "Spectrometer_Close" {
            n187 = Unbundle By Name(w495) -> ("Abstract_CCD.lvclass"=w498:refnum<class "Abstract_CCD.lvclass">)
            n188 = flat-sequence {
              tunnel: [refnum<class "Abstract_CCD.lvclass"> refnum ("Abstract_CCD.lvclass")] -> w492
              tunnel: w491 -> [_]
              frame #0 {
              }
            }
            n189 = call-dynamic "Close.vi"("error in (no error)"=w497, "Abstract_CCD in"=w498) -> ("error out"=w491:errorcluster)  [unwired: 8 in, 1 out]
            n190 = Bundle By Name(cluster=w495, "Abstract_CCD.lvclass"=w492) -> (w494:T3)
          }
          frame "Spectrometer_Measure" {
            w512 = T4 {"QueueAction"=enum."TimeOut", "Data"=[], "Data_Raw"=[], "Data_Dark"=[], "Data_Ref"=[], "Device Information"=[], "Numeric Control"=0.0, "Boolean"=FALSE, "Wavelength"=[], "Time"=[], "Time Stamp"=timestamp(0 s since 1904-01-01)}  # DataQueue
            n191 = Unbundle By Name(w507) -> ("Abstract_CCD.lvclass"=w511:refnum<class "Abstract_CCD.lvclass">)
            n192 = call-dynamic "Measure.vi"("error in (no error)"=w509, "Abstract_CCD in"=w511) -> ("error out"=w508:errorcluster, "Data Raw"=w502:T8, "Data"=w503:T8, "Darkspec"=w501:T8, "Time"=w500:dbl[])  [unwired: 3 in, 2 out]
            n193 = Bundle By Name(cluster=w512, "QueueAction"=DataQueue_Action."TimeOut", "Data"=w503, "Data_Raw"=w502, "Data_Dark"=w501, "Time"=w500) -> (w513:T4)
            n194 = Enqueue Element(queue=w506, element=w513) -> (queue out=w505:refnum<queue>)  [unwired: 2 in, 2 out]
          }
          frame "Spectrometer_Preview" {
            w528 = T4 {"QueueAction"=enum."TimeOut", "Data"=[], "Data_Raw"=[], "Data_Dark"=[], "Data_Ref"=[], "Device Information"=[], "Numeric Control"=0.0, "Boolean"=FALSE, "Wavelength"=[], "Time"=[], "Time Stamp"=timestamp(0 s since 1904-01-01)}  # DataQueue
            n195 = Unbundle By Name(w516) -> ("Abstract_CCD.lvclass"=w533:refnum<class "Abstract_CCD.lvclass">)
            n196 = call-dynamic "Get_Frames.vi"("error in (no error)"=w532, "Abstract_CCD in"=w533) -> ("error out"=w534:errorcluster, "Numeric"=w520:i32, "Abstract_CCD out"=w535:refnum<class "Abstract_CCD.lvclass">)  [unwired: 7 in]
            n197 = call-dynamic "Set_Frames.vi"("error in (no error)"=w534, "Frames"=1, "Abstract_CCD in"=w535) -> ("error out"=w531:errorcluster, "Abstract_CCD out"=w536:refnum<class "Abstract_CCD.lvclass">)  [unwired: 7 in]
            n198 = call-dynamic "Measure.vi"("error in (no error)"=w531, "Abstract_CCD in"=w536) -> ("error out"=w522:errorcluster, "Data Raw"=w525:T8, "Abstract_CCD out"=w521:refnum<class "Abstract_CCD.lvclass">)  [unwired: 3 in, 4 out]
            n199 = property on="Preview" class="Bool (strict)"() -> ("Value"=w523:bool)  [unwired: 2 in, 2 out]
            n200 = call-dynamic "Set_Frames.vi"("error in (no error)"=w522, "Frames"=w520, "Abstract_CCD in"=w521) -> ("error out"=w519:errorcluster, "Abstract_CCD out"=w514:refnum<class "Abstract_CCD.lvclass">)  [unwired: 7 in]
            n201 = case shown="True" w523 {
              tunnel: [w537 w539] -> w518
              tunnel: w517 -> [w537 w538]
              frame False {
              }
              frame True {
                w541 = T6 {"QueueAction"=enum."TimeOut", "Numeric 1"=0.0, "Numeric 2"=0.0, "Boolean 1"=FALSE, "Boolean 2"=FALSE, "Spin Program"=[]}  # Device Queue
                n202 = Bundle By Name(cluster=w541, "QueueAction"=DeviceQueue_Action."Spectrometer_Preview") -> (w540:T6)
                n203 = Enqueue Element(queue=w538, element=w540) -> (queue out=w539:refnum<queue>)  [unwired: 2 in, 2 out]
              }
            }
            n204 = Bundle By Name(cluster=w528, "Data_Raw"=w525, "QueueAction"=DataQueue_Action."Spectrometer_Measure") -> (w529:T4)
            n205 = Enqueue Element(queue=w527, element=w529) -> (queue out=w526:refnum<queue>)  [unwired: 2 in, 2 out]
            n206 = Bundle By Name(cluster=w516, "Abstract_CCD.lvclass"=w514) -> (w515:T3)
          }
          frame "Spectrometer_SetIntegrationTime" {
            n207 = Unbundle By Name(w551) -> ("Numeric 1"=w553:dbl)
            n208 = Unbundle By Name(w545) -> ("Abstract_CCD.lvclass"=w555:refnum<class "Abstract_CCD.lvclass">)
            n209 = Unbundle By Name(w551) -> ("Boolean 1"=w550:bool)
            n210 = node(w553) -> (w552:dbl[unit])
            n211 = call-dynamic "Set_ExposureTime.vi"("error in (no error)"=w554, "Exposure Time"=w552, "Abstract_CCD in"=w555) -> ("error out"=w558:errorcluster, "Abstract_CCD out"=w557:refnum<class "Abstract_CCD.lvclass">)  [unwired: 7 in]
            n212 = call-dynamic "Get_FrameRate.vi"("error in (no error)"=w558, "Abstract_CCD in"=w557) -> ("error out"=w546:errorcluster, "Frame Rate"=w549:dbl[unit], "Abstract_CCD out"=w544:refnum<class "Abstract_CCD.lvclass">)  [unwired: 7 in]
            "Frame Rate" <- w549
            n213 = Bundle By Name(cluster=w545, "Abstract_CCD.lvclass"=w544) -> (w543:T3)
            n214 = case shown="True" w550 {
              tunnel: w549 -> [_ w567]
              tunnel: w548 -> [w559 w561]
              tunnel: [w559 w560] -> w547
              frame False {
              }
              frame True {
                w565 = T6 {"QueueAction"=enum."TimeOut", "Numeric 1"=0.0, "Numeric 2"=0.0, "Boolean 1"=FALSE, "Boolean 2"=FALSE, "Spin Program"=[]}  # Device Queue
                n215 = property on="Program Spin Coater\nSpeed (rpm)          Time (s)" class="Arr (strict)"() -> ("Value"=w570:dbl[][])  [unwired: 2 in, 2 out]
                n216 = property on="Seconds to Spin Start" class="DigNum (strict)"() -> ("Value"=w569:dbl[unit])  [unwired: 2 in, 2 out]
                n217 = property on="Seconds after Spin Stop" class="DigNum (strict)"() -> ("Value"=w568:dbl[unit])  [unwired: 2 in, 2 out]
                n218 = call "CalculateFrames.vi"("Program Spin Coater\nSpeed (rpm)          Time (s)"=w570, "Seconds End"=w568, "Seconds Start"=w569, "Frame Rate"=w567) -> ("Time"=w566:dbl, "Frames"=w562:i32)  [unwired: 6 in]
                n219 = property on="Overall Time" class="DigNum (strict)"("Value"=w566) -> ()  [unwired: 2 in, 2 out]
                n220 = Bundle By Name(cluster=w565, "QueueAction"=DeviceQueue_Action."Spectrometer_SetFrames", "Numeric 1"=w562) -> (w564:T6)
                n221 = Enqueue Element(queue=w561, element=w564) -> (queue out=w560:refnum<queue>)  [unwired: 2 in, 2 out]
              }
            }
          }
          frame "Spectrometer_SetFrames" {
            n222 = Unbundle By Name(w572) -> ("Abstract_CCD.lvclass"=w577:refnum<class "Abstract_CCD.lvclass">)
            n223 = Unbundle By Name(w580) -> ("Numeric 1"=w574:dbl)
            n224 = property on="Frames" class="DigNum (strict)"("Value"=w574) -> ()  [unwired: 2 in, 2 out]
            n225 = call-dynamic "Set_Frames.vi"("error in (no error)"=w576, "Frames"=w574, "Abstract_CCD in"=w577) -> ("error out"=w575:errorcluster, "Abstract_CCD out"=w571:refnum<class "Abstract_CCD.lvclass">)  [unwired: 7 in]
            n226 = Bundle By Name(cluster=w572, "Abstract_CCD.lvclass"=w571) -> (w573:T3)
          }
          frame "Spectrometer_SetDarkspec" {
            w588 = T4 {"QueueAction"=enum."TimeOut", "Data"=[], "Data_Raw"=[], "Data_Dark"=[], "Data_Ref"=[], "Device Information"=[], "Numeric Control"=0.0, "Boolean"=FALSE, "Wavelength"=[], "Time"=[], "Time Stamp"=timestamp(0 s since 1904-01-01)}  # DataQueue
            n227 = Unbundle By Name(w583) -> ("Abstract_CCD.lvclass"=w600:refnum<class "Abstract_CCD.lvclass">)
            n228 = property on="Frames for Dark/Ref" class="DigNum (strict)"() -> ("Value"=w590:dbl)  [unwired: 2 in, 2 out]
            n229 = call-dynamic "Get_Frames.vi"("error in (no error)"=w592, "Abstract_CCD in"=w600) -> ("error out"=w597:errorcluster, "Numeric"=w598:i32, "Abstract_CCD out"=w599:refnum<class "Abstract_CCD.lvclass">)  [unwired: 7 in]
            n230 = call-dynamic "Set_Frames.vi"("error in (no error)"=w597, "Frames"=w590, "Abstract_CCD in"=w599) -> ("error out"=w596:errorcluster, "Abstract_CCD out"=w593:refnum<class "Abstract_CCD.lvclass">)  [unwired: 7 in]
            n231 = call-dynamic "Measure.vi"("error in (no error)"=w596, "Abstract_CCD in"=w593) -> ("error out"=w595:errorcluster, "Data Raw"=w585:T8, "Abstract_CCD out"=w594:refnum<class "Abstract_CCD.lvclass">)  [unwired: 3 in, 4 out]
            n232 = call-dynamic "Set_Frames.vi"("error in (no error)"=w595, "Frames"=w598, "Abstract_CCD in"=w594) -> ("error out"=w591:errorcluster, "Abstract_CCD out"=w581:refnum<class "Abstract_CCD.lvclass">)  [unwired: 7 in]
            n233 = Bundle By Name(cluster=w588, "QueueAction"=DataQueue_Action."Set_Dark", "Data_Dark"=w585) -> (w589:T4)
            n234 = Enqueue Element(queue=w587, element=w589) -> (queue out=w584:refnum<queue>)  [unwired: 2 in, 2 out]
            n235 = Bundle By Name(cluster=w583, "Abstract_CCD.lvclass"=w581) -> (w582:T3)
          }
          frame "Spectrometer_SetReference" {
            w609 = T4 {"QueueAction"=enum."TimeOut", "Data"=[], "Data_Raw"=[], "Data_Dark"=[], "Data_Ref"=[], "Device Information"=[], "Numeric Control"=0.0, "Boolean"=FALSE, "Wavelength"=[], "Time"=[], "Time Stamp"=timestamp(0 s since 1904-01-01)}  # DataQueue
            n236 = Unbundle By Name(w604) -> ("Abstract_CCD.lvclass"=w621:refnum<class "Abstract_CCD.lvclass">)
            n237 = property on="Frames for Dark/Ref" class="DigNum (strict)"() -> ("Value"=w611:dbl)  [unwired: 2 in, 2 out]
            n238 = call-dynamic "Get_Frames.vi"("error in (no error)"=w613, "Abstract_CCD in"=w621) -> ("error out"=w618:errorcluster, "Numeric"=w619:i32, "Abstract_CCD out"=w620:refnum<class "Abstract_CCD.lvclass">)  [unwired: 7 in]
            n239 = call-dynamic "Set_Frames.vi"("error in (no error)"=w618, "Frames"=w611, "Abstract_CCD in"=w620) -> ("error out"=w617:errorcluster, "Abstract_CCD out"=w614:refnum<class "Abstract_CCD.lvclass">)  [unwired: 7 in]
            n240 = call-dynamic "Measure.vi"("error in (no error)"=w617, "Abstract_CCD in"=w614) -> ("error out"=w616:errorcluster, "Data Raw"=w606:T8, "Abstract_CCD out"=w615:refnum<class "Abstract_CCD.lvclass">)  [unwired: 3 in, 4 out]
            n241 = call-dynamic "Set_Frames.vi"("error in (no error)"=w616, "Frames"=w619, "Abstract_CCD in"=w615) -> ("error out"=w612:errorcluster, "Abstract_CCD out"=w602:refnum<class "Abstract_CCD.lvclass">)  [unwired: 7 in]
            n242 = Bundle By Name(cluster=w609, "QueueAction"=DataQueue_Action."Set_Ref", "Data_Ref"=w606) -> (w610:T4)
            n243 = Enqueue Element(queue=w608, element=w610) -> (queue out=w605:refnum<queue>)  [unwired: 2 in, 2 out]
            n244 = Bundle By Name(cluster=w604, "Abstract_CCD.lvclass"=w602) -> (w603:T3)
          }
          frame "Arduino_Init" {
            w634 = T6 {"QueueAction"=enum."TimeOut", "Numeric 1"=0.0, "Numeric 2"=0.0, "Boolean 1"=FALSE, "Boolean 2"=FALSE, "Spin Program"=[]}  # Device Queue
            n245 = call-poly "VISA Configure Serial Port"("VISA resource name"="Port Arduino", "baud rate (9600)"=u32 115200, "error in (no error)"=w640) -> ("VISA resource name out"=w636:refnum<visa-resource-name>, "error out"=w632:errorcluster)  [unwired: 11 in]
            n246 = property on="Program Spin Coater\nSpeed (rpm)          Time (s)" class="Arr (strict)"() -> ("Value"=w628:dbl[][])  [unwired: 2 in, 2 out]
            n247 = Bundle By Name(cluster=w634, "QueueAction"=DeviceQueue_Action."Arduino_LoadProgram", "Spin Program"=dbl[][] []) -> (w629:T6)
            n248 = Enqueue Element(queue=w631, element=w629, error in (no error)=w632) -> (queue out=w627:refnum<queue>, error out=w626:errorcluster)  [unwired: 1 in, 1 out]
            n249 = Bundle By Name(cluster=w629, "Spin Program"=w628) -> (w625:T6)
            n250 = Bundle By Name(cluster=w637, "Port Arduino"=w636) -> (w635:T3)
            n251 = Enqueue Element(queue=w627, element=w625, error in (no error)=w626) -> (queue out=w624:refnum<queue>, error out=w623:errorcluster)  [unwired: 1 in, 1 out]
          }
          frame "Arduino_Close" {
            n252 = Unbundle By Name(w643) -> ("Port Arduino"=w647:refnum<visa-resource-name>)
            n253 = VISA Close(VISA resource name=w647, error in (no error)=w646) -> (error out=w645:errorcluster)
          }
          frame "Arduino_LoadProgram" {
            n254 = Unbundle By Name(w650) -> ("Spin Program"=w649:dbl[][])
            n255 = Unbundle By Name(w652) -> ("Port Arduino"=w654:refnum<visa-resource-name>)
            n256 = call "SpinCoaterArray2String.vi"("Program Spin Coater\nSpeed (rpm)          Time (s)"=w649) -> ("remote control String"=w648:string)  [unwired: 4 in]
            n257 = VISA Write(VISA resource name=w654, write buffer=w648, error in (no error)=w655) -> (error out=w651:errorcluster)  [unwired: 2 out]
          }
          frame "Arduino_StartProgram" {
            n258 = Unbundle By Name(w662) -> ("Port Arduino"=w661:refnum<visa-resource-name>)
            n259 = VISA Write(VISA resource name=w661, write buffer="run", error in (no error)=w659) -> (error out=w658:errorcluster)  [unwired: 2 out]
          }
          frame "Arduino_SetSpeed" {
            n260 = Unbundle By Name(w672) -> ("Numeric 1"=w670:dbl)
            n261 = Unbundle By Name(w674) -> ("Port Arduino"=w673:refnum<visa-resource-name>)
            n262 = To Unsigned Long Integer(number=w670) -> (unsigned 32bit integer=w669:u32)
            n263 = Number To Decimal String(number=w669) -> (decimal integer string=w668:string)  [unwired: 1 in]
            n264 = Concatenate Strings("!spe" ("string"), w668) -> (w666:string)
            n265 = VISA Write(VISA resource name=w673, write buffer=w666, error in (no error)=w671) -> (error out=w665:errorcluster)  [unwired: 2 out]
          }
          frame "Arduino_SetMillis" {
            n266 = Unbundle By Name(w678) -> ("Numeric 1"=w686:dbl)
            n267 = Unbundle By Name(w676) -> ("Port Arduino"=w687:refnum<visa-resource-name>)
            n268 = To Unsigned Long Integer(number=w686) -> (unsigned 32bit integer=w685:u32)
            n269 = Number To Decimal String(number=w685) -> (decimal integer string=w684:string)  [unwired: 1 in]
            n270 = Concatenate Strings("!mil" ("string"), w684) -> (w682:string)
            n271 = VISA Write(VISA resource name=w687, write buffer=w682, error in (no error)=w681) -> (error out=w679:errorcluster)  [unwired: 2 out]
          }
          frame "Arduino_StopSpin" {
            n272 = Unbundle By Name(w691) -> ("Port Arduino"=w690:refnum<visa-resource-name>)
            n273 = VISA Write(VISA resource name=w690, write buffer="abo", error in (no error)=w692) -> (error out=w688:errorcluster)  [unwired: 2 out]
          }
          frame "Measure_InSitu" {
            w702 = T4 {"QueueAction"=enum."TimeOut", "Data"=[], "Data_Raw"=[], "Data_Dark"=[], "Data_Ref"=[], "Device Information"=[], "Numeric Control"=0.0, "Boolean"=FALSE, "Wavelength"=[], "Time"=[], "Time Stamp"=timestamp(0 s since 1904-01-01)}  # DataQueue
            n274 = flat-sequence {
              tunnel: w704 -> [w724]
              tunnel: [w723] -> w717
              tunnel: [w722] -> w716
              tunnel: [w721] -> w714
              tunnel: w709 -> [w720]
              tunnel: [w720] -> w711
              tunnel: w717 -> [w727]
              tunnel: w716 -> [w725]
              tunnel: [w729] -> w715
              tunnel: w714 -> [w728]
              tunnel: [w728] -> w713
              tunnel: [w727] -> w712
              tunnel: w711 -> [w726]
              tunnel: [w726] -> w710
              tunnel: [w725] -> w708
              tunnel: w715 -> [_]
              tunnel: w713 -> [w745]
              tunnel: w712 -> [w744]
              tunnel: w710 -> [w741]
              tunnel: w708 -> [w743]
              tunnel: [w738] -> w699
              tunnel: [w737] -> w700
              tunnel: [w736] -> w707
              tunnel: [w735] -> w705
              tunnel: [w734] -> w701
              frame #0 {
                n275 = Unbundle By Name(w724) -> ("Abstract_CCD.lvclass"=w723:refnum<class "Abstract_CCD.lvclass">, "Port Arduino"=w722:refnum<visa-resource-name>)
                n276 = property on="Seconds to Spin Start" class="DigNum (strict)"() -> ("Value"=w719:dbl[unit])  [unwired: 2 in, 2 out]
                n277 = node(w719) -> (w721:dbl)
              }
              frame #1 {
                n278 = call <vilib>:"High Resolution Relative Seconds.vi"() -> ("relative seconds"=w729:dbl)
              }
              frame #2 {
                n279 = flat-sequence {
                  tunnel: w745 -> [w747]
                  tunnel: w741 -> [w746]
                  tunnel: [w746] -> w742
                  tunnel: w743 -> [w752]
                  tunnel: w742 -> [w750]
                  tunnel: [w749] -> w739
                  tunnel: [w748] -> w735
                  frame #0 {
                    n280 = Wait (ms)(milliseconds to wait=w747) -> ()  [unwired: 1 out]
                  }
                  frame #1 {
                    n281 = call <vilib>:"High Resolution Relative Seconds.vi"() -> ("relative seconds"=w749:dbl)
                    n282 = VISA Write(VISA resource name=w752, write buffer="run", error in (no error)=w750) -> (error out=w748:errorcluster)  [unwired: 2 out]
                  }
                }
                n283 = flat-sequence {
                  tunnel: w744 -> [w758]
                  tunnel: w741 -> [w757]
                  tunnel: [w756] -> w733
                  tunnel: [w755] -> w732
                  tunnel: [w754] -> w731
                  tunnel: [w753] -> w730
                  tunnel: [w760] -> w738
                  tunnel: [w761] -> w737
                  tunnel: [w762] -> w736
                  tunnel: [w763] -> w740
                  tunnel: w733 -> [w763]
                  tunnel: w732 -> [w762]
                  tunnel: w731 -> [w761]
                  tunnel: w730 -> [w760]
                  frame #0 {
                    n284 = call-dynamic "Measure.vi"("error in (no error)"=w757, "Abstract_CCD in"=w758) -> ("error out"=w755:errorcluster, "Data Raw"=w754:T8, "Time"=w753:dbl[], "Starting Time"=w756:dbl)  [unwired: 3 in, 3 out]
                  }
                  frame #1 {
                    n285 = property on="StartMeasurement_Button" class="Bool (strict)"("Value"=FALSE ("StartMeasurement_Button")) -> ()  [unwired: 2 in, 2 out]
                  }
                }
                n286 = Subtract(x=w740, y=w739) -> (x-y=w734:dbl)
              }
            }
            n287 = property on="Action" class="Str"("Value"="Measuring" ("Action")) -> ()  [unwired: 2 in, 2 out]
            n288 = Bundle By Name(cluster=w702, "Time"=w699, "Data_Raw"=w700, "Numeric Control"=w701, "QueueAction"=DataQueue_Action."Measure_InSituSpinCoating") -> (w703:T4)
            n289 = Merge Errors(w707, w705) -> (w706:errorcluster)
            n290 = Enqueue Element(queue=w697, element=w703) -> (queue out=w696:refnum<queue>)  [unwired: 2 in, 2 out]
          }
        }
      }
      frame Error {
        w768 = T11 4 items=["no dialog", "OK message", "continue or stop message", "OK message + warnings", "continue/stop + warnings"] ("type of dialog (OK msg:1)")
        n291 = call <vilib>:"General Error Handler.vi"("type of dialog (OK msg:1)"=w768, "error in (no error)"=w769) -> ("error out"=w767:errorcluster)  [unwired: 9 in, 4 out]
        n292 = call <vilib>:"Clear Errors.vi"("error in (no error)"=w767) -> ("error out"=w766:errorcluster)  [unwired: 5 in, 1 out]
      }
    }
  }
  n293 = Release Queue(queue=w4) -> ()  [unwired: 2 in, 3 out]
  n294 = Release Queue(queue=w5) -> ()  [unwired: 2 in, 3 out]
